vi "Motors Bk 3.vi"(0 "Set":refnum<vi>, 3 "Enable Motors":refnum<vi>, 4 "Scan in Progress":refnum<vi>, 8 "Cluster":T1, 11 "Motors Visa Ref":refnum<visa-resource-name>="COM7") -> ()   [LabVIEW 2010]
uses:
  <vilib>/Utility/error.llb/DialogType.ctl
panel:
  in  "Set Backlash":bool
  out "Motors error":refnum<vi>
  out "theta-":refnum<vi>
  out "theta+":refnum<vi>
  out "Delta Theta (deg)":refnum<vi>
  out "Theta Speed (deg/s)":refnum<vi>
  out "theta-?":refnum<vi>
  out "theta+?":refnum<vi>
  out "Defined Positions":refnum<vi>
  out "Go To Saved Position?":refnum<vi>
  out "Saved Positions":refnum<vi>
  out "z-":refnum<vi>
  out "z+":refnum<vi>
  out "Delta Z (mm)":refnum<vi>
  out "Z Speed (mm/s)":refnum<vi>
  out "z-?":refnum<vi>
  out "z+?":refnum<vi>
  out "Y Speed (mm/s)":refnum<vi>
  out "y-":refnum<vi>
  out "y+":refnum<vi>
  out "Delta Y (mm)":refnum<vi>
  out "y-?":refnum<vi>
  out "y+?":refnum<vi>
  out "x-":refnum<vi>
  out "x+":refnum<vi>
  out "X Speed (mm/s)":refnum<vi>
  out "Delta X (mm)":refnum<vi>
  out "x-?":refnum<vi>
  out "x+?":refnum<vi>
  out "Jog-Mode":refnum<vi>
  out "Theta Go To":refnum<vi>
  out "Theta Go?":refnum<vi>
  out "Z Go To":refnum<vi>
  out "Z Go?":refnum<vi>
  out "Y Go To":refnum<vi>
  out "Y Go?":refnum<vi>
  out "X Go To":refnum<vi>
  out "X Go?":refnum<vi>
  out "Use Datums Nearest Hard Limits to Reset Origin?":refnum<vi>
  out "Saved Limits":refnum<vi>
  out "Find Datums Nearest Hard Limits?":refnum<vi>
  out "Theta Moving":refnum<vi>
  out "Status Theta":refnum<vi>
  out "Theta (deg)":refnum<vi>
  out "Theta Jogger Fast Speed":refnum<vi>
  out "Theta Jogger Normal Speed":refnum<vi>
  out "Theta Slew Speed (mm or degree/s)":refnum<vi>
  out "Z Moving":refnum<vi>
  out "Status Z":refnum<vi>
  out "Z-Axis (mm)":refnum<vi>
  out "Z Jogger Fast Speed":refnum<vi>
  out "Z Jogger Normal Speed":refnum<vi>
  out "Z Slew Speed (mm or degree/s)":refnum<vi>
  out "Y Moving":refnum<vi>
  out "Status Y":refnum<vi>
  out "Y-Axis (mm)":refnum<vi>
  out "Y Jogger Fast Speed":refnum<vi>
  out "Y Jogger Normal Speed":refnum<vi>
  out "Y Slew Speed (mm or degree/s)":refnum<vi>
  out "X Moving":refnum<vi>
  out "Status X":refnum<vi>
  out "X-Axis (mm)":refnum<vi>
  out "X Slew Speed (mm or degree/s)":refnum<vi>
  out "X Jogger Fast Speed":refnum<vi>
  out "X Jogger Normal Speed":refnum<vi>
  out "Set Jogger?":refnum<vi>
  out "Normal":refnum<vi>
  out "Fast":refnum<vi>
  out "Jogger Axis":refnum<vi>
  out "Theta Multiplier":refnum<vi>
  out "Z Multiplier":refnum<vi>
  out "Y Multiplier":refnum<vi>
  out "X Multiplier":refnum<vi>
  out "Need to Update Motor Parameters":refnum<vi>
  out "(degrees/s)":refnum<vi>
  out "Theta Set Slew Speed?":refnum<vi>
  out "(mm/s) 3":refnum<vi>
  out "Z Set Slew Speed?":refnum<vi>
  out "(mm/s) 2":refnum<vi>
  out "Y Set Slew Speed?":refnum<vi>
  out "(mm/s)":refnum<vi>
  out "X Set Slew Speed?":refnum<vi>
  out "Save Current Motor Parameters?":refnum<vi>
  out "Redefine Origin as Current Location?":refnum<vi>
  out "Reset Motors?":refnum<vi>
  out "Manual Communication is Active\n(Close Before Ending Program)":refnum<vi>
  out "Manual IO?":refnum<vi>
  out "EMERGENCY":refnum<vi>
  out "Backlash Theta":refnum<vi>
  out "Backlash Z":refnum<vi>
  out "Backlash Y":refnum<vi>
  out "Backlash X":refnum<vi>
  out "Backlash?":refnum<vi>
  out "Stop Theta?":refnum<vi>
  out "Stop Z?":refnum<vi>
  out "Stop Y?":refnum<vi>
  out "Stop X?":refnum<vi>
  out "Theta Action":string
  out "Z Action":string
  out "Y Action":string
  out "X Action":string
  in  "Steps to deactivate hard limit after finding datums":dbl=1000.0
  out "Loop i":i32
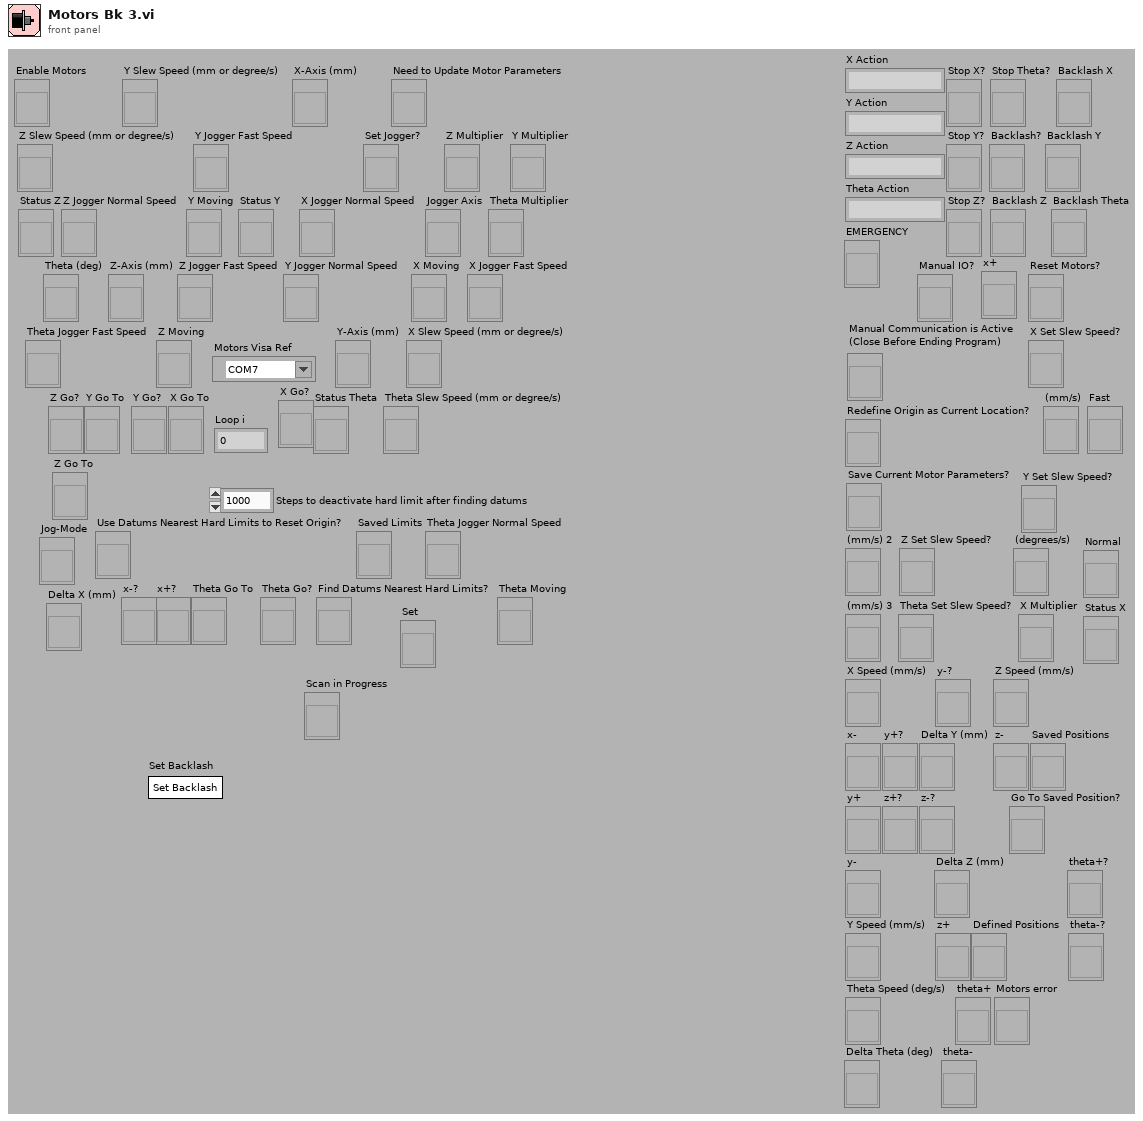
[diagram p1: front panel]
types:
  T1 = cluster{"Stop X?":refnum<vi>, "Stop Y?":refnum<vi>, "Stop Z?":refnum<vi>, "Stop Theta?":refnum<vi>, "Backlash?":refnum<vi>, "Backlash X":refnum<vi>, "Backlash Y":refnum<vi>, "Backlash Z":refnum<vi>, "Backlash Theta":refnum<vi>, "Manual IO?":refnum<vi>, "Manual Communication is Active\n(Close Before Ending Program)":refnum<vi>, "Reset Motors?":refnum<vi>, "Set Jogger?":refnum<vi>, "Normal":refnum<vi>, "Fast":refnum<vi>, "Jogger Axis":refnum<vi>, "Redefine Origin as Current Location?":refnum<vi>, "Save Current Motor Parameters?":refnum<vi>, "Find Datums Nearest Hard Limits?":refnum<vi>, "Saved Limits":refnum<vi>, "Use Datums Nearest Hard Limits to Reset Origin?":refnum<vi>, "X Go?":refnum<vi>, "Y Go?":refnum<vi>, "Z Go?":refnum<vi>, "Theta Go?":refnum<vi>, "Jog-Mode":refnum<vi>, "x+?":refnum<vi>, "x-?":refnum<vi>, "y+?":refnum<vi>, "y-?":refnum<vi>, "z+?":refnum<vi>, "z-?":refnum<vi>, "theta+?":refnum<vi>, "theta-?":refnum<vi>, "X Set Slew Speed?":refnum<vi>, "(mm/s)":refnum<vi>, "Y Set Slew Speed?":refnum<vi>, "(mm/s)":refnum<vi>, "Z Set Slew Speed?":refnum<vi>, "(mm/s)":refnum<vi>, "Theta Set Slew Speed?":refnum<vi>, "(degrees/s)":refnum<vi>, "Go To Saved Position?":refnum<vi>, "Defined Positions":refnum<vi>, "Need to Update Motor Parameters":refnum<vi>, "X Jogger Normal Speed":refnum<vi>, "X Jogger Fast Speed":refnum<vi>, "Y Jogger Normal Speed":refnum<vi>, "Y Jogger Fast Speed":refnum<vi>, "Z Jogger Normal Speed":refnum<vi>, "Z Jogger Fast Speed":refnum<vi>, "Theta Jogger Normal Speed":refnum<vi>, "Theta Jogger Fast Speed":refnum<vi>, "X Moving":refnum<vi>, "Y Moving":refnum<vi>, "Z Moving":refnum<vi>, "Theta Moving":refnum<vi>, "X Slew Speed (mm or degree/s)":refnum<vi>, "Y Slew Speed (mm or degree/s)":refnum<vi>, "Z Slew Speed (mm or degree/s)":refnum<vi>, "Theta Slew Speed (mm or degree/s)":refnum<vi>, "X-Axis (mm)":refnum<vi>, "Y-Axis (mm)":refnum<vi>, "Z-Axis (mm)":refnum<vi>, "Theta (deg)":refnum<vi>, "X Multiplier":refnum<vi>, "Y Multiplier":refnum<vi>, "Z Multiplier":refnum<vi>, "Theta Multiplier":refnum<vi>, "Motors Online":refnum<vi>, "Motors Status":refnum<vi>, "Status X":refnum<vi>, "Status Y":refnum<vi>, "Status Z":refnum<vi>, "Status Theta":refnum<vi>, "Motors error":refnum<vi>, "QUIT":refnum<vi>, "EMERGENCY":refnum<vi>, "X Go To":refnum<vi>, "Y Go To":refnum<vi>, "Z Go To":refnum<vi>, "Theta Go To":refnum<vi>, "Delta X (mm)":refnum<vi>, "Delta Y (mm)":refnum<vi>, "Delta Z (mm)":refnum<vi>, "Delta Theta (deg)":refnum<vi>, "X Speed (mm/s)":refnum<vi>, "Y Speed (mm/s)":refnum<vi>, "Z Speed (mm/s)":refnum<vi>, "Theta Speed (deg/s)":refnum<vi>, "x+":refnum<vi>, "x-":refnum<vi>, "y+":refnum<vi>, "y-":refnum<vi>, "z+":refnum<vi>, "z-":refnum<vi>, "theta+":refnum<vi>, "theta-":refnum<vi>, "Saved Positions":refnum<vi>}
  T2 = typedef "DialogType.ctl" = u16
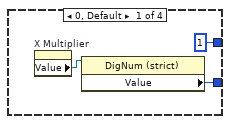
[diagram p4: hidden frame]
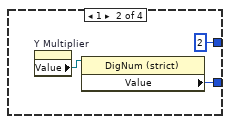
[diagram p5: hidden frame]
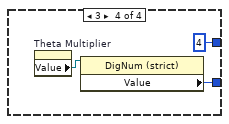
[diagram p6: hidden frame]
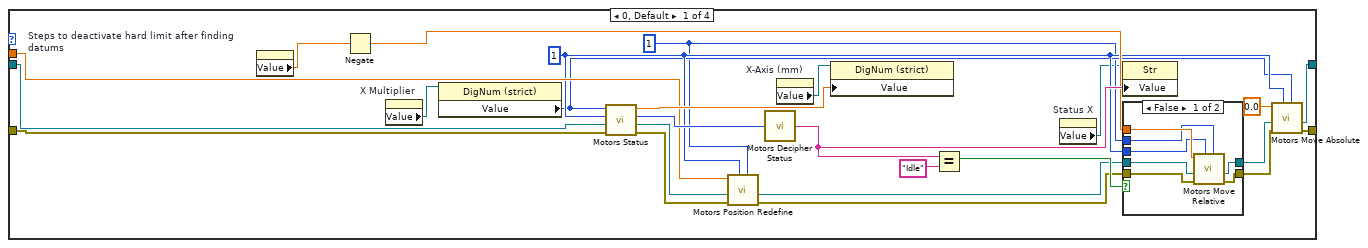
[diagram p16: hidden frame]
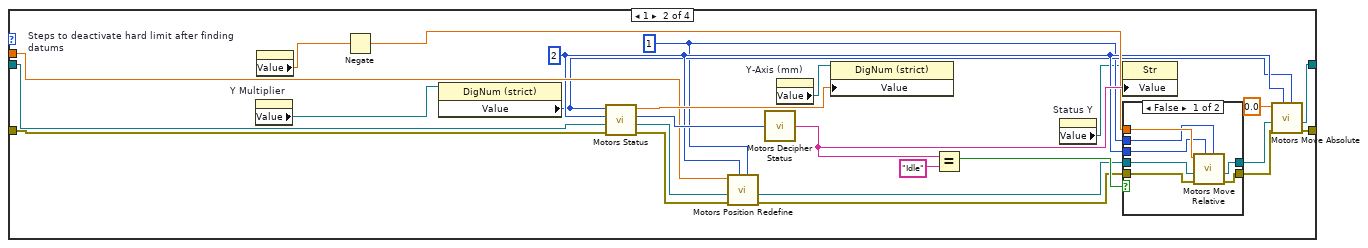
[diagram p18: hidden frame]
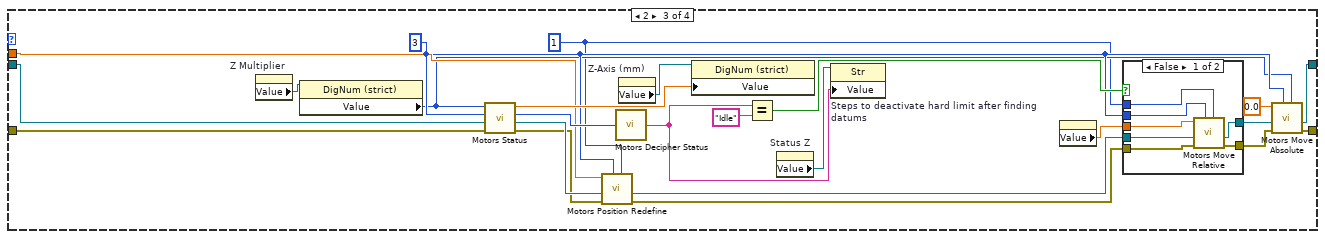
[diagram p20: hidden frame]
diagram:
  w2 = T2 0 items=["no dialog", "OK message", "continue or stop message", "OK message + warnings", "continue/stop + warnings"] ("type of dialog (OK msg:1)")
  n1 = call "Motors Open.vi"("VISA in"="Motors Visa Ref") -> ("error out"=w112:errorcluster, "VISA out"=w4:refnum<visa-resource-name>)  [unwired: 1 in]
  n2 = call <vilib>:"Simple Error Handler.vi"("type of dialog (OK msg:1)"=w2, "error in (no error)"=w112) -> ("error?"=w111:bool, "error out"=w113:errorcluster)  [unwired: 3 in, 3 out]
  n3 = Unbundle("Cluster") -> ("Stop X?"=→"Stop X?":refnum<vi>, "Stop Y?"=→"Stop Y?":refnum<vi>, "Stop Z?"=→"Stop Z?":refnum<vi>, "Stop Theta?"=→"Stop Theta?":refnum<vi>, "Backlash?"=→"Backlash?":refnum<vi>, "Backlash X"=→"Backlash X":refnum<vi>, "Backlash Y"=→"Backlash Y":refnum<vi>, "Backlash Z"=→"Backlash Z":refnum<vi>, "Backlash Theta"=→"Backlash Theta":refnum<vi>, "Manual IO?"=→"Manual IO?":refnum<vi>, "Manual Communication is Active\n(Close Before Ending Program)"=→"Manual Communication is Active\n(Close Before Ending Program)":refnum<vi>, "Reset Motors?"=→"Reset Motors?":refnum<vi>, "Set Jogger?"=→"Set Jogger?":refnum<vi>, "Normal"=→"Normal":refnum<vi>, "Fast"=→"Fast":refnum<vi>, "Jogger Axis"=→"Jogger Axis":refnum<vi>, "Redefine Origin as Current Location?"=→"Redefine Origin as Current Location?":refnum<vi>, "Save Current Motor Parameters?"=→"Save Current Motor Parameters?":refnum<vi>, "Find Datums Nearest Hard Limits?"=→"Find Datums Nearest Hard Limits?":refnum<vi>, "Saved Limits"=→"Saved Limits":refnum<vi>, "Use Datums Nearest Hard Limits to Reset Origin?"=→"Use Datums Nearest Hard Limits to Reset Origin?":refnum<vi>, "X Go?"=→"X Go?":refnum<vi>, "Y Go?"=→"Y Go?":refnum<vi>, "Z Go?"=→"Z Go?":refnum<vi>, "Theta Go?"=→"Theta Go?":refnum<vi>, "Jog-Mode"=→"Jog-Mode":refnum<vi>, "x+?"=→"x+?":refnum<vi>, "x-?"=→"x-?":refnum<vi>, "y+?"=→"y+?":refnum<vi>, "y-?"=→"y-?":refnum<vi>, "z+?"=→"z+?":refnum<vi>, "z-?"=→"z-?":refnum<vi>, "theta+?"=→"theta+?":refnum<vi>, "theta-?"=→"theta-?":refnum<vi>, "X Set Slew Speed?"=→"X Set Slew Speed?":refnum<vi>, "(mm/s)"=→"(mm/s)":refnum<vi>, "Y Set Slew Speed?"=→"Y Set Slew Speed?":refnum<vi>, "(mm/s)"=→"(mm/s) 2":refnum<vi>, "Z Set Slew Speed?"=→"Z Set Slew Speed?":refnum<vi>, "(mm/s)"=→"(mm/s) 3":refnum<vi>, "Theta Set Slew Speed?"=→"Theta Set Slew Speed?":refnum<vi>, "(degrees/s)"=→"(degrees/s)":refnum<vi>, "Go To Saved Position?"=→"Go To Saved Position?":refnum<vi>, "Defined Positions"=→"Defined Positions":refnum<vi>, "Need to Update Motor Parameters"=w7:refnum<vi>, "X Jogger Normal Speed"=→"X Jogger Normal Speed":refnum<vi>, "X Jogger Fast Speed"=→"X Jogger Fast Speed":refnum<vi>, "Y Jogger Normal Speed"=→"Y Jogger Normal Speed":refnum<vi>, "Y Jogger Fast Speed"=→"Y Jogger Fast Speed":refnum<vi>, "Z Jogger Normal Speed"=→"Z Jogger Normal Speed":refnum<vi>, "Z Jogger Fast Speed"=→"Z Jogger Fast Speed":refnum<vi>, "Theta Jogger Normal Speed"=→"Theta Jogger Normal Speed":refnum<vi>, "Theta Jogger Fast Speed"=→"Theta Jogger Fast Speed":refnum<vi>, "X Moving"=→"X Moving":refnum<vi>, "Y Moving"=→"Y Moving":refnum<vi>, "Z Moving"=→"Z Moving":refnum<vi>, "Theta Moving"=→"Theta Moving":refnum<vi>, "X Slew Speed (mm or degree/s)"=→"X Slew Speed (mm or degree/s)":refnum<vi>, "Y Slew Speed (mm or degree/s)"=→"Y Slew Speed (mm or degree/s)":refnum<vi>, "Z Slew Speed (mm or degree/s)"=→"Z Slew Speed (mm or degree/s)":refnum<vi>, "Theta Slew Speed (mm or degree/s)"=→"Theta Slew Speed (mm or degree/s)":refnum<vi>, "X-Axis (mm)"=→"X-Axis (mm)":refnum<vi>, "Y-Axis (mm)"=→"Y-Axis (mm)":refnum<vi>, "Z-Axis (mm)"=→"Z-Axis (mm)":refnum<vi>, "Theta (deg)"=→"Theta (deg)":refnum<vi>, "X Multiplier"=→"X Multiplier":refnum<vi>, "Y Multiplier"=→"Y Multiplier":refnum<vi>, "Z Multiplier"=→"Z Multiplier":refnum<vi>, "Theta Multiplier"=→"Theta Multiplier":refnum<vi>, "Motors Online"=w89:refnum<vi>, "Motors Status"=w90:refnum<vi>, "Status X"=→"Status X":refnum<vi>, "Status Y"=→"Status Y":refnum<vi>, "Status Z"=→"Status Z":refnum<vi>, "Status Theta"=→"Status Theta":refnum<vi>, "Motors error"=w1:refnum<vi>, "QUIT"=w109:refnum<vi>, "EMERGENCY"=→"EMERGENCY":refnum<vi>, "X Go To"=→"X Go To":refnum<vi>, "Y Go To"=→"Y Go To":refnum<vi>, "Z Go To"=→"Z Go To":refnum<vi>, "Theta Go To"=→"Theta Go To":refnum<vi>, "Delta X (mm)"=→"Delta X (mm)":refnum<vi>, "Delta Y (mm)"=→"Delta Y (mm)":refnum<vi>, "Delta Z (mm)"=→"Delta Z (mm)":refnum<vi>, "Delta Theta (deg)"=→"Delta Theta (deg)":refnum<vi>, "X Speed (mm/s)"=→"X Speed (mm/s)":refnum<vi>, "Y Speed (mm/s)"=→"Y Speed (mm/s)":refnum<vi>, "Z Speed (mm/s)"=→"Z Speed (mm/s)":refnum<vi>, "Theta Speed (deg/s)"=→"Theta Speed (deg/s)":refnum<vi>, "x+"=→"x+":refnum<vi>, "x-"=→"x-":refnum<vi>, "y+"=→"y+":refnum<vi>, "y-"=→"y-":refnum<vi>, "z+"=→"z+":refnum<vi>, "z-"=→"z-":refnum<vi>, "theta+"=→"theta+":refnum<vi>, "theta-"=→"theta-":refnum<vi>, "Saved Positions"=→"Saved Positions":refnum<vi>)
  "Need to Update Motor Parameters" <- w7
  "Motors error" <- w1
  n4 = property on="Property Node" class="Clust (strict)"(reference=w1, "Value"=w113) -> ()  [unwired: 1 in, 2 out]
  n5 = property on="Property Node" class="Bool (strict)"(reference=w7, "Value"=TRUE) -> ()  [unwired: 1 in, 2 out]
  n6 = Not(x=w111) -> (.not. x?=w110:bool)
  n7 = property on="Property Node" class="Bool (strict)"(reference=w89, "Value"=w110) -> ()  [unwired: 1 in, 2 out]
  n8 = property on="Property Node" class="Str"(reference=w90, "Value"="Opening Communication Channels") -> (reference out=w108:refnum<vi>)  [unwired: 1 in, 1 out]
  n9 = case shown="True" w110 {
    tunnel: w108 -> [_ w121]
    tunnel: w4 -> [w115 w120]
    tunnel: w1 -> [_ w119]
    tunnel: w109 -> [_ w118]
    tunnel: [w115 w116] -> w3
    frame False {
    }
    frame True {
      n10 = property on="Property Node" class="Str"(reference=w121, "Value"="Running") -> (reference out=w117:refnum<vi>)  [unwired: 1 in, 1 out]
      n11 = while {
        shift-right: [w132] -> w116
        shift-left: w120 -> [w138]
        tunnel: w119 -> [w137]
        tunnel: w118 -> [w140]
        tunnel: w117 -> [w139]
        i -> [w141]
        stop <- w123 stop-if-true
        n12 = property on="Property Node" class="Bool (strict)"(reference="Enable Motors") -> ("Value"=w134:bool)  [unwired: 1 in, 2 out]
        n13 = property on="Property Node" class="Bool (strict)"(reference=w140) -> ("Value"=w136:bool)  [unwired: 1 in, 2 out]
        n14 = property on="Property Node" class="Bool (strict)"(reference="Set") -> (reference out=w126:refnum<vi>, "Value"=w129:bool)  [unwired: 1 in, 1 out]
        n15 = property on="Property Node" class="Bool (strict)"(reference="Scan in Progress") -> ("Value"=w125:bool)  [unwired: 1 in, 2 out]
        n16 = Not(x=w134) -> (.not. x?=w133:bool)
        n17 = Or(x=w136, y=w133) -> (x .or. y?=w124:bool)
        n18 = Or(x=w124, y=w125) -> (x .or. y?=w123:bool)
        n19 = Not(x=w125) -> (.not. x?=w127:bool)
        n20 = Or(x=w129, y=w127) -> (x .or. y?=w131:bool)
        n21 = case shown="True" w131 {
          tunnel: w141 -> [_ w263]
          tunnel: w139 -> [_ w260]
          tunnel: w138 -> [w142 w226]
          tunnel: w137 -> [_ w184]
          tunnel: [w142 w145] -> w132
          tunnel: w126 -> [_ w144]
          frame False {
          }
          frame True {
            # "This loop contains all of the code that has to communicate directly with the manipulator motor controllers.  They are arranged linearly to ensure multiple serial I/O's are never attempted simultaneously.  Note that this loop executes very slowly (each serial I/O takes about 1/20 sec).\n\nWarning: Pushing LabView's \"Clean Up Diagram\" button will likely cause LabView to crash (because this VI is way too big)."
            n22 = property on="Stop X?" class="LVObjRef (strict)"() -> ("Value"=w183:refnum<vi>)  [unwired: 2 in, 2 out]
            n23 = property on="Reset Motors?" class="LVObjRef (strict)"() -> ("Value"=w177:refnum<vi>)  [unwired: 2 in, 2 out]
            n24 = property on="Property Node" class="Bool (strict)"(reference=w144, "Value"=FALSE) -> ()  [unwired: 1 in, 2 out]
            n25 = property on="Property Node" class="Bool (strict)"(reference=w183) -> (reference out=w240:refnum<vi>, "Value"=w233:bool)  [unwired: 1 in, 1 out]
            n26 = property on="Property Node" class="Bool (strict)"(reference=w177) -> (reference out=w220:refnum<vi>, "Value"=w219:bool)  [unwired: 1 in, 1 out]
            n27 = property on="Property Node" class="Clust (strict)"(reference=w184) -> (reference out=w147:refnum<vi>, "Value"=w225:errorcluster)  [unwired: 1 in, 1 out]
            n28 = case shown="True" w233 {
              tunnel: w225 -> [w417 w425]
              tunnel: w226 -> [w418 w424]
              tunnel: [w418 w422] -> w232
              tunnel: [w417 w421] -> w231
              tunnel: w240 -> [_ w419]
              frame False {
              }
              frame True {
                n29 = property on="Property Node" class="Bool (strict)"(reference=w419, "Value"=FALSE) -> ()  [unwired: 1 in, 2 out]
                n30 = call "Motors Stop.vi"("error in"=w425, "Axis"=1, "VISA in"=w424) -> ("error out"=w421:errorcluster, "VISA out"=w422:refnum<visa-resource-name>)
              }
            }
            n31 = property on="Stop Y?" class="LVObjRef (strict)"() -> ("Value"=w182:refnum<vi>)  [unwired: 2 in, 2 out]
            n32 = property on="Property Node" class="Bool (strict)"(reference=w182) -> (reference out=w239:refnum<vi>, "Value"=w234:bool)  [unwired: 1 in, 1 out]
            n33 = case shown="True" w234 {
              tunnel: w231 -> [w408 w416]
              tunnel: w232 -> [w409 w415]
              tunnel: [w409 w413] -> w230
              tunnel: [w408 w412] -> w229
              tunnel: w239 -> [_ w410]
              frame False {
              }
              frame True {
                n34 = property on="Property Node" class="Bool (strict)"(reference=w410, "Value"=FALSE) -> ()  [unwired: 1 in, 2 out]
                n35 = call "Motors Stop.vi"("error in"=w416, "Axis"=2, "VISA in"=w415) -> ("error out"=w412:errorcluster, "VISA out"=w413:refnum<visa-resource-name>)
              }
            }
            n36 = property on="Stop Z?" class="LVObjRef (strict)"() -> ("Value"=w181:refnum<vi>)  [unwired: 2 in, 2 out]
            n37 = property on="Property Node" class="Bool (strict)"(reference=w181) -> (reference out=w238:refnum<vi>, "Value"=w235:bool)  [unwired: 1 in, 1 out]
            n38 = case shown="True" w235 {
              tunnel: w229 -> [w399 w407]
              tunnel: w230 -> [w400 w406]
              tunnel: [w400 w404] -> w228
              tunnel: [w399 w403] -> w227
              tunnel: w238 -> [_ w401]
              frame False {
              }
              frame True {
                n39 = property on="Property Node" class="Bool (strict)"(reference=w401, "Value"=FALSE) -> ()  [unwired: 1 in, 2 out]
                n40 = call "Motors Stop.vi"("error in"=w407, "Axis"=3, "VISA in"=w406) -> ("error out"=w403:errorcluster, "VISA out"=w404:refnum<visa-resource-name>)
              }
            }
            n41 = property on="Stop Theta?" class="LVObjRef (strict)"() -> ("Value"=w180:refnum<vi>)  [unwired: 2 in, 2 out]
            n42 = property on="Property Node" class="Bool (strict)"(reference=w180) -> (reference out=w237:refnum<vi>, "Value"=w236:bool)  [unwired: 1 in, 1 out]
            n43 = case shown="True" w236 {
              tunnel: w227 -> [w390 w398]
              tunnel: w228 -> [w391 w397]
              tunnel: [w391 w395] -> w221
              tunnel: [w390 w394] -> w222
              tunnel: w237 -> [_ w392]
              frame False {
              }
              frame True {
                n44 = property on="Property Node" class="Bool (strict)"(reference=w392, "Value"=FALSE) -> ()  [unwired: 1 in, 2 out]
                n45 = call "Motors Stop.vi"("error in"=w398, "Axis"=4, "VISA in"=w397) -> ("error out"=w394:errorcluster, "VISA out"=w395:refnum<visa-resource-name>)
              }
            }
            n46 = property on="Backlash?" class="LVObjRef (strict)"() -> ("Value"=w179:refnum<vi>)  [unwired: 2 in, 2 out]
            n47 = property on="Property Node" class="Bool (strict)"(reference=w179) -> (reference out=w224:refnum<vi>, "Value"=w223:bool)  [unwired: 1 in, 1 out]
            n48 = case shown="True" w223 {
              tunnel: [w375 w389] -> w214
              tunnel: w224 -> [_ w383]
              tunnel: w221 -> [w375 w382]
              tunnel: w222 -> [w374 w381]
              tunnel: [w374 w380] -> w213
              frame False {
              }
              frame True {
                n49 = property on="Property Node" class="Bool (strict)"(reference=w383, "Value"=FALSE) -> ()  [unwired: 1 in, 2 out]
                n50 = property on="Backlash X" class="LVObjRef (strict)"() -> ("Value"=w379:refnum<vi>)  [unwired: 2 in, 2 out]
                n51 = property on="Backlash Z" class="LVObjRef (strict)"() -> ("Value"=w377:refnum<vi>)  [unwired: 2 in, 2 out]
                n52 = property on="Backlash Y" class="LVObjRef (strict)"() -> ("Value"=w378:refnum<vi>)  [unwired: 2 in, 2 out]
                n53 = property on="Backlash Theta" class="LVObjRef (strict)"() -> ("Value"=w376:refnum<vi>)  [unwired: 2 in, 2 out]
                n54 = property on="Property Node" class="DigNum (strict)"(reference=w379) -> ("Value"=w388:u32)  [unwired: 1 in, 2 out]
                n55 = property on="Property Node" class="DigNum (strict)"(reference=w376) -> ("Value"=w385:u32)  [unwired: 1 in, 2 out]
                n56 = property on="Property Node" class="DigNum (strict)"(reference=w377) -> ("Value"=w386:u32)  [unwired: 1 in, 2 out]
                n57 = property on="Property Node" class="DigNum (strict)"(reference=w378) -> ("Value"=w387:u32)  [unwired: 1 in, 2 out]
                n58 = call "Motors Backlash.vi"("X"=w388, "Y"=w387, "VISA in"=w382, "error in"=w381, "Z"=w386, "Theta"=w385) -> ("VISA out"=w389:refnum<visa-resource-name>, "error out"=w380:errorcluster)  [unwired: 2 in]
              }
            }
            n59 = property on="Manual IO?" class="LVObjRef (strict)"() -> ("Value"=w178:refnum<vi>)  [unwired: 2 in, 2 out]
            n60 = property on="Property Node" class="Bool (strict)"(reference=w178) -> (reference out=w218:refnum<vi>, "Value"=w217:bool)  [unwired: 1 in, 1 out]
            n61 = case shown="True" w217 {
              tunnel: [w349 w360] -> w216
              tunnel: [w350 w352] -> w215
              tunnel: w218 -> [_ w354]
              tunnel: w214 -> [w350 w353]
              tunnel: w213 -> [w349 w351]
              frame False {
              }
              frame True {
                n62 = flat-sequence {
                  tunnel: [w362] -> w356
                  tunnel: [w369] -> w359
                  tunnel: [w368] -> w358
                  tunnel: [w367] -> w357
                  tunnel: w356 -> [w367]
                  tunnel: w353 -> [w366]
                  tunnel: w351 -> [w365]
                  tunnel: [w372] -> w352
                  tunnel: [w373] -> w360
                  tunnel: w359 -> [w373]
                  tunnel: w358 -> [w372]
                  tunnel: w357 -> [w370]
                  frame #0 {
                    n63 = property on="Manual Communication is Active\n(Close Before Ending Program)" class="LVObjRef (strict)"() -> ("Value"=w361:refnum<vi>)  [unwired: 2 in, 2 out]
                    n64 = property on="Property Node" class="Bool (strict)"(reference=w361, "Value"=TRUE ("Manual Communication is Active\n(Close Before Ending Program) 2")) -> (reference out=w362:refnum<vi>)  [unwired: 1 in, 1 out]
                  }
                  frame #1 {
                    n65 = property on="EMERGENCY" class="LVObjRef (strict)"() -> ("Value"=w364:refnum<vi>)  [unwired: 2 in, 2 out]
                    n66 = call "Motors Manual IO.vi"("error in"=w365, "Emergency Stop Reference"=w364, "VISA in"=w366) -> ("error out"=w369:errorcluster, "VISA out"=w368:refnum<visa-resource-name>)
                  }
                  frame #2 {
                    n67 = property on="Property Node" class="Bool (strict)"(reference=w370, "Value"=FALSE ("Manual Communication is Active\n(Close Before Ending Program)")) -> ()  [unwired: 1 in, 2 out]
                  }
                }
                n68 = property on="Property Node" class="Bool (strict)"(reference=w354, "Value"=FALSE) -> ()  [unwired: 1 in, 2 out]
              }
            }
            n69 = property on="Jogger Axis" class="LVObjRef (strict)"() -> ("Value"=w169:refnum<vi>)  [unwired: 2 in, 2 out]
            n70 = property on="Property Node" class="Ring (strict)"(reference=w169) -> ("Value"=w212:u16)  [unwired: 1 in, 2 out]
            n71 = case shown="2" w212 {
              tunnel: [u32 1 u32 2 u32 3 u32 4] -> _
              tunnel: [w315 w318 w321 w324] -> w211
              frame 0, Default {
                n72 = property on="X Multiplier" class="LVObjRef (strict)"() -> ("Value"=w314:refnum<vi>)  [unwired: 2 in, 2 out]
                n73 = property on="Property Node" class="DigNum (strict)"(reference=w314) -> ("Value"=w315:u32)  [unwired: 1 in, 2 out]
              }
              frame 1 {
                n74 = property on="Y Multiplier" class="LVObjRef (strict)"() -> ("Value"=w317:refnum<vi>)  [unwired: 2 in, 2 out]
                n75 = property on="Property Node" class="DigNum (strict)"(reference=w317) -> ("Value"=w318:u32)  [unwired: 1 in, 2 out]
              }
              frame 2 {
                n76 = property on="Z Multiplier" class="LVObjRef (strict)"() -> ("Value"=w320:refnum<vi>)  [unwired: 2 in, 2 out]
                n77 = property on="Property Node" class="DigNum (strict)"(reference=w320) -> ("Value"=w321:u32)  [unwired: 1 in, 2 out]
              }
              frame 3 {
                n78 = property on="Theta Multiplier" class="LVObjRef (strict)"() -> ("Value"=w323:refnum<vi>)  [unwired: 2 in, 2 out]
                n79 = property on="Property Node" class="DigNum (strict)"(reference=w323) -> ("Value"=w324:u32)  [unwired: 1 in, 2 out]
              }
            }
            n80 = case shown="True" w219 {
              tunnel: [w341 w348] -> w207
              tunnel: [w342 w347] -> w208
              tunnel: w215 -> [w342 w346]
              tunnel: w216 -> [w341 w345]
              tunnel: w220 -> [_ w343]
              frame False {
              }
              frame True {
                n81 = property on="Property Node" class="Bool (strict)"(reference=w343, "Value"=FALSE) -> ()  [unwired: 1 in, 2 out]
                n82 = call "Motors Reset.vi"("error in"=w345, "VISA in"=w346) -> ("error out"=w348:errorcluster, "VISA out"=w347:refnum<visa-resource-name>)
              }
            }
            n83 = property on="Set Jogger?" class="LVObjRef (strict)"() -> ("Value"=w170:refnum<vi>)  [unwired: 2 in, 2 out]
            n84 = property on="Property Node" class="Bool (strict)"(reference=w170) -> (reference out=w210:refnum<vi>, "Value"=w209:bool)  [unwired: 1 in, 1 out]
            n85 = case shown="True" w209 {
              tunnel: [w327 w340] -> w205
              tunnel: [w326 w338] -> w206
              tunnel: w211 -> [_ w339]
              tunnel: w210 -> [_ w336]
              tunnel: w207 -> [w327 w332]
              tunnel: w208 -> [w326 w331]
              frame False {
              }
              frame True {
                n86 = property on="Property Node" class="Bool (strict)"(reference=w336, "Value"=FALSE ("Need to Update Motor Parameters")) -> ()  [unwired: 1 in, 2 out]
                n87 = property on="Normal" class="LVObjRef (strict)"() -> ("Value"=w329:refnum<vi>)  [unwired: 2 in, 2 out]
                n88 = property on="Need to Update Motor Parameters" class="LVObjRef (strict)"() -> ("Value"=w328:refnum<vi>)  [unwired: 2 in, 2 out]
                n89 = property on="Fast" class="LVObjRef (strict)"() -> ("Value"=w330:refnum<vi>)  [unwired: 2 in, 2 out]
                n90 = property on="Property Node" class="DigNum (strict)"(reference=w329) -> ("Value"=w335:dbl)  [unwired: 1 in, 2 out]
                n91 = property on="Property Node" class="DigNum (strict)"(reference=w330) -> ("Value"=w334:dbl)  [unwired: 1 in, 2 out]
                n92 = property on="Property Node" class="Bool (strict)"(reference=w328, "Value"=TRUE) -> ()  [unwired: 1 in, 2 out]
                n93 = call "Motors Jogger Speed.vi"("Axis Multiplier"=w339, "error in"=w332, "VISA in"=w331, "Fast Speed (mm or degree/sec)"=w334, "Normal Speed (mm or degree/sec)"=w335) -> ("error out"=w340:errorcluster, "VISA out"=w338:refnum<visa-resource-name>)  [unwired: 5 in]
              }
            }
            n94 = property on="Redefine Origin as Current Location?" class="LVObjRef (strict)"() -> ("Value"=w176:refnum<vi>)  [unwired: 2 in, 2 out]
            n95 = property on="Property Node" class="Bool (strict)"(reference=w176) -> (reference out=w252:refnum<vi>, "Value"=w262:bool)  [unwired: 1 in, 1 out]
            n96 = case shown="True" w262 {
              tunnel: w206 -> [w1424 w1431]
              tunnel: w205 -> [w1425 w1427]
              tunnel: [w1425 w1429] -> w255
              tunnel: [w1424 w1430] -> w313
              tunnel: w252 -> [_ w1426]
              frame False {
              }
              frame True {
                n97 = property on="Property Node" class="Bool (strict)"(reference=w1426, "Value"=FALSE) -> ()  [unwired: 1 in, 2 out]
                n98 = call "Motors Redefine Origin.vi"("error in"=w1427, "VISA in"=w1431) -> ("error out"=w1429:errorcluster, "VISA out"=w1430:refnum<visa-resource-name>)
              }
            }
            n99 = property on="Save Current Motor Parameters?" class="LVObjRef (strict)"() -> ("Value"=w175:refnum<vi>)  [unwired: 2 in, 2 out]
            n100 = property on="Property Node" class="Bool (strict)"(reference=w175) -> (reference out=w254:refnum<vi>, "Value"=w253:bool)  [unwired: 1 in, 1 out]
            n101 = case shown="True" w253 {
              tunnel: w255 -> [w1417 w1423]
              tunnel: [w1417 w1422] -> w269
              tunnel: w313 -> [w1416 w1421]
              tunnel: [w1416 w1420] -> w268
              tunnel: w254 -> [_ w1419]
              frame False {
              }
              frame True {
                n102 = property on="Property Node" class="Bool (strict)"(reference=w1419, "Value"=FALSE) -> ()  [unwired: 1 in, 2 out]
                n103 = call "Motors Save.vi"("error in"=w1423, "VISA in"=w1421) -> ("error out"=w1422:errorcluster, "VISA out"=w1420:refnum<visa-resource-name>)
              }
            }
            n104 = property on="Find Datums Nearest Hard Limits?" class="LVObjRef (strict)"() -> ("Value"=w167:refnum<vi>)  [unwired: 2 in, 2 out]
            n105 = property on="Property Node" class="Bool (strict)"(reference=w167) -> (reference out=w256:refnum<vi>, "Value"=w261:bool)  [unwired: 1 in, 1 out]
            n106 = case shown="True" w261 {
              tunnel: w269 -> [w605 w618]
              tunnel: [w605 w616] -> w266
              tunnel: [w604 w617] -> w264
              tunnel: w268 -> [w604 w619]
              tunnel: w260 -> [w603 w611]
              tunnel: [w603 w608] -> w258
              tunnel: w256 -> [_ w607]
              frame False {
              }
              frame True {
                n107 = property on="Property Node" class="Bool (strict)"(reference=w607, "Value"=FALSE) -> ()  [unwired: 1 in, 2 out]
                n108 = flat-sequence {
                  tunnel: w618 -> [w624]
                  tunnel: w619 -> [w625]
                  tunnel: [w625] -> w615
                  tunnel: [w624] -> w614
                  tunnel: w611 -> [w621]
                  tunnel: [w620] -> w609
                  tunnel: w615 -> [w644]
                  tunnel: w614 -> [w643]
                  tunnel: [w639] -> w613
                  tunnel: [w638] -> w612
                  tunnel: [w628] -> w610
                  tunnel: w609 -> [w628]
                  tunnel: [w738] -> w616
                  tunnel: [w739] -> w617
                  tunnel: w613 -> [w739]
                  tunnel: w612 -> [w738]
                  tunnel: w610 -> [w736]
                  tunnel: [w735] -> w608
                  frame #0 {
                    n109 = call <vilib>:"Set Busy.vi"("disable click? (T)"=FALSE) -> ()  [unwired: 9 in, 2 out]
                    n110 = property on="Property Node" class="Str"(reference=w621, "Value"="Finding Datums Nearest Hard Limits\nThis May Take a Few Minutes" ("Status")) -> (reference out=w620:refnum<vi>)  [unwired: 1 in, 1 out]
                  }
                  frame #1 {
                    n111 = call "Motors Find Datums.vi"("error in"=w643, "VISA in"=w644) -> ("error out"=w640:errorcluster, "VISA out"=w641:refnum<visa-resource-name>)
                    n112 = for {
                      N: 4 -> [_]
                      shift-right: [w648] -> w638
                      shift-left: w640 -> [w649]
                      shift-right: [w647] -> w639
                      shift-left: w641 -> [w650]
                      tunnel: [w646] -> w630 mode=indexing
                      i -> [w645]
                      n113 = case shown="3" w645 {
                        tunnel: w649 -> [w663 w684 w705 w726]
                        tunnel: w650 -> [w664 w685 w706 w727]
                        tunnel: [w657 w678 w698 w719] -> w648
                        tunnel: [w658 w679 w699 w720] -> w647
                        tunnel: [w655 w676 w702 w723] -> w646
                        frame 0, Default {
                          w656 = 1 ("Axis")
                          n114 = property on="X Multiplier" class="LVObjRef (strict)"() -> ("Value"=w651:refnum<vi>)  [unwired: 2 in, 2 out]
                          n115 = property on="Property Node" class="DigNum (strict)"(reference=w651) -> ("Value"=w662:u32)  [unwired: 1 in, 2 out]
                          n116 = call "Motors Status.vi"("error in"=w663, "VISA in"=w664, "Axis"=w656, "Axis Multiplier"=w662) -> ("error out"=w659:errorcluster, "VISA out"=w660:refnum<visa-resource-name>, "OS"=w669:i32, "Actual Position (mm or deg)"=w661:dbl)  [unwired: 3 in]
                          n117 = call "Motors Datum Position.vi"("error in"=w659, "VISA in"=w660, "Axis"=w656) -> ("error out"=w657:errorcluster, "VISA out"=w658:refnum<visa-resource-name>, "Datum Position (steps)"=w655:string)  [unwired: 5 in]
                          n118 = call "Motors Decipher Status.vi"("OS"=w669) -> ("Status"=w668:string)
                          n119 = property on="X-Axis (mm)" class="LVObjRef (strict)"() -> ("Value"=w653:refnum<vi>)  [unwired: 2 in, 2 out]
                          n120 = property on="Property Node" class="DigNum (strict)"(reference=w653, "Value"=w661) -> ()  [unwired: 1 in, 2 out]
                          n121 = Equal?(x=w668, y="Idle") -> (x = y?=w666:bool)
                          n122 = property on="Status X" class="LVObjRef (strict)"() -> ("Value"=w654:refnum<vi>)  [unwired: 2 in, 2 out]
                          n123 = case shown="False" w666 {
                            tunnel: [TRUE FALSE] -> w665
                            frame False {
                            }
                            frame True {
                            }
                          }
                          n124 = property on="Property Node" class="Str"(reference=w654, "Value"=w668) -> ()  [unwired: 1 in, 2 out]
                          n125 = property on="X Moving" class="LVObjRef (strict)"() -> ("Value"=w652:refnum<vi>)  [unwired: 2 in, 2 out]
                          n126 = property on="Property Node" class="Bool (strict)"(reference=w652, "Value"=w665) -> ()  [unwired: 1 in, 2 out]
                        }
                        frame 1 {
                          w677 = 2 ("Axis")
                          n127 = property on="Y Multiplier" class="LVObjRef (strict)"() -> ("Value"=w675:refnum<vi>)  [unwired: 2 in, 2 out]
                          n128 = property on="Property Node" class="DigNum (strict)"(reference=w675) -> ("Value"=w683:u32)  [unwired: 1 in, 2 out]
                          n129 = call "Motors Status.vi"("error in"=w684, "VISA in"=w685, "Axis"=w677, "Axis Multiplier"=w683) -> ("error out"=w680:errorcluster, "VISA out"=w681:refnum<visa-resource-name>, "OS"=w690:i32, "Actual Position (mm or deg)"=w682:dbl)  [unwired: 3 in]
                          n130 = call "Motors Datum Position.vi"("error in"=w680, "VISA in"=w681, "Axis"=w677) -> ("error out"=w678:errorcluster, "VISA out"=w679:refnum<visa-resource-name>, "Datum Position (steps)"=w676:string)  [unwired: 5 in]
                          n131 = call "Motors Decipher Status.vi"("OS"=w690) -> ("Status"=w688:string)
                          n132 = property on="Y-Axis (mm)" class="LVObjRef (strict)"() -> ("Value"=w672:refnum<vi>)  [unwired: 2 in, 2 out]
                          n133 = property on="Property Node" class="DigNum (strict)"(reference=w672, "Value"=w682) -> ()  [unwired: 1 in, 2 out]
                          n134 = Equal?(x=w688, y="Idle") -> (x = y?=w687:bool)
                          n135 = property on="Status Y" class="LVObjRef (strict)"() -> ("Value"=w674:refnum<vi>)  [unwired: 2 in, 2 out]
                          n136 = case shown="False" w687 {
                            tunnel: [TRUE FALSE] -> w686
                            frame False {
                            }
                            frame True {
                            }
                          }
                          n137 = property on="Property Node" class="Str"(reference=w674, "Value"=w688) -> ()  [unwired: 1 in, 2 out]
                          n138 = property on="Y Moving" class="LVObjRef (strict)"() -> ("Value"=w673:refnum<vi>)  [unwired: 2 in, 2 out]
                          n139 = property on="Property Node" class="Bool (strict)"(reference=w673, "Value"=w686) -> ()  [unwired: 1 in, 2 out]
                        }
                        frame 2 {
                          w697 = 3 ("Axis")
                          n140 = property on="Z Multiplier" class="LVObjRef (strict)"() -> ("Value"=w696:refnum<vi>)  [unwired: 2 in, 2 out]
                          n141 = property on="Property Node" class="DigNum (strict)"(reference=w696) -> ("Value"=w704:u32)  [unwired: 1 in, 2 out]
                          n142 = call "Motors Status.vi"("error in"=w705, "VISA in"=w706, "Axis"=w697, "Axis Multiplier"=w704) -> ("error out"=w700:errorcluster, "VISA out"=w701:refnum<visa-resource-name>, "OS"=w711:i32, "Actual Position (mm or deg)"=w703:dbl)  [unwired: 3 in]
                          n143 = call "Motors Datum Position.vi"("error in"=w700, "VISA in"=w701, "Axis"=w697) -> ("error out"=w698:errorcluster, "VISA out"=w699:refnum<visa-resource-name>, "Datum Position (steps)"=w702:string)  [unwired: 5 in]
                          n144 = call "Motors Decipher Status.vi"("OS"=w711) -> ("Status"=w709:string)
                          n145 = property on="Z-Axis (mm)" class="LVObjRef (strict)"() -> ("Value"=w693:refnum<vi>)  [unwired: 2 in, 2 out]
                          n146 = property on="Property Node" class="DigNum (strict)"(reference=w693, "Value"=w703) -> ()  [unwired: 1 in, 2 out]
                          n147 = Equal?(x=w709, y="Idle") -> (x = y?=w708:bool)
                          n148 = property on="Status Z" class="LVObjRef (strict)"() -> ("Value"=w695:refnum<vi>)  [unwired: 2 in, 2 out]
                          n149 = case shown="False" w708 {
                            tunnel: [TRUE FALSE] -> w707
                            frame False {
                            }
                            frame True {
                            }
                          }
                          n150 = property on="Property Node" class="Str"(reference=w695, "Value"=w709) -> ()  [unwired: 1 in, 2 out]
                          n151 = property on="Z Moving" class="LVObjRef (strict)"() -> ("Value"=w694:refnum<vi>)  [unwired: 2 in, 2 out]
                          n152 = property on="Property Node" class="Bool (strict)"(reference=w694, "Value"=w707) -> ()  [unwired: 1 in, 2 out]
                        }
                        frame 3 {
                          w718 = 4 ("Axis")
                          n153 = property on="Theta Multiplier" class="LVObjRef (strict)"() -> ("Value"=w716:refnum<vi>)  [unwired: 2 in, 2 out]
                          n154 = property on="Property Node" class="DigNum (strict)"(reference=w716) -> ("Value"=w725:u32)  [unwired: 1 in, 2 out]
                          n155 = call "Motors Status.vi"("error in"=w726, "VISA in"=w727, "Axis"=w718, "Axis Multiplier"=w725) -> ("error out"=w721:errorcluster, "VISA out"=w722:refnum<visa-resource-name>, "OS"=w732:i32, "Actual Position (mm or deg)"=w724:dbl)  [unwired: 3 in]
                          n156 = call "Motors Datum Position.vi"("error in"=w721, "VISA in"=w722, "Axis"=w718) -> ("error out"=w719:errorcluster, "VISA out"=w720:refnum<visa-resource-name>, "Datum Position (steps)"=w723:string)  [unwired: 5 in]
                          n157 = call "Motors Decipher Status.vi"("OS"=w732) -> ("Status"=w730:string)
                          n158 = property on="Theta (deg)" class="LVObjRef (strict)"() -> ("Value"=w717:refnum<vi>)  [unwired: 2 in, 2 out]
                          n159 = property on="Property Node" class="DigNum (strict)"(reference=w717, "Value"=w724) -> ()  [unwired: 1 in, 2 out]
                          n160 = Equal?(x=w730, y="Idle") -> (x = y?=w729:bool)
                          n161 = property on="Status Theta" class="LVObjRef (strict)"() -> ("Value"=w715:refnum<vi>)  [unwired: 2 in, 2 out]
                          n162 = case shown="True" w729 {
                            tunnel: [TRUE FALSE] -> w728
                            frame False {
                            }
                            frame True {
                            }
                          }
                          n163 = property on="Property Node" class="Str"(reference=w715, "Value"=w730) -> ()  [unwired: 1 in, 2 out]
                          n164 = property on="Theta Moving" class="LVObjRef (strict)"() -> ("Value"=w714:refnum<vi>)  [unwired: 2 in, 2 out]
                          n165 = property on="Property Node" class="Bool (strict)"(reference=w714, "Value"=w728) -> ()  [unwired: 1 in, 2 out]
                        }
                      }
                    }
                    n166 = Build Array (concatenate)("Limits", w630) -> (w629:string[])
                    n167 = Initialize Array("", 0 ("dimension size"), 0 ("dimension size")) -> (w636:string[][])
                    n168 = Build Array (concatenate)(w629, w636) -> (w634:string[][])
                    n169 = property on="Saved Limits" class="LVObjRef (strict)"() -> ("Value"=w626:refnum<vi>)  [unwired: 2 in, 2 out]
                    n170 = property on="Property Node" class="Path"(reference=w626) -> ("Value"=w627:path)  [unwired: 1 in, 2 out]
                    n171 = Transpose 2D Array(2D array=w634) -> (transposed array=w633:string[][])
                    n172 = call "Motors Position Rewrite.vi"("file path"=w627, "Array of Positions"=w633) -> ()  [unwired: 9 in]
                  }
                  frame #2 {
                    n173 = call <vilib>:"Unset Busy.vi"() -> ()  [unwired: 11 in, 1 out]
                    n174 = property on="Property Node" class="Str"(reference=w736, "Value"="Running" ("Status")) -> (reference out=w735:refnum<vi>)  [unwired: 1 in, 1 out]
                  }
                }
              }
            }
            n175 = property on="Use Datums Nearest Hard Limits to Reset Origin?" class="LVObjRef (strict)"() -> ("Value"=w166:refnum<vi>)  [unwired: 2 in, 2 out]
            n176 = property on="Property Node" class="Bool (strict)"(reference=w166) -> (reference out=w146:refnum<vi>, "Value"=w259:bool)  [unwired: 1 in, 1 out]
            n177 = case shown="True" w259 {
              tunnel: [w428 w436] -> w267
              tunnel: w266 -> [w428 w438]
              tunnel: [w427 w435] -> w265
              tunnel: w264 -> [w427 w439]
              tunnel: w258 -> [w426 w431]
              tunnel: [w426 w432] -> w186
              tunnel: w146 -> [_ w430]
              frame False {
              }
              frame True {
                n178 = property on="Property Node" class="Bool (strict)"(reference=w430, "Value"=FALSE) -> ()  [unwired: 1 in, 2 out]
                n179 = flat-sequence {
                  tunnel: w438 -> [w443]
                  tunnel: [w443] -> w437
                  tunnel: w431 -> [w441]
                  tunnel: [w440] -> w433
                  tunnel: w439 -> [w455]
                  tunnel: w437 -> [w456]
                  tunnel: [w451] -> w436
                  tunnel: [w450] -> w435
                  tunnel: [w445] -> w434
                  tunnel: w433 -> [w445]
                  tunnel: w434 -> [w601]
                  tunnel: [w600] -> w432
                  frame #0 {
                    n180 = call <vilib>:"Set Busy.vi"() -> ()  [unwired: 10 in, 2 out]
                    n181 = property on="Property Node" class="Str"(reference=w441, "Value"="Finding Datums Nearest Hard Limits\nThis May Take a Few Minutes" ("Status")) -> (reference out=w440:refnum<vi>)  [unwired: 1 in, 1 out]
                  }
                  frame #1 {
                    n182 = property on="Saved Limits" class="LVObjRef (strict)"() -> ("Value"=w444:refnum<vi>)  [unwired: 2 in, 2 out]
                    n183 = property on="Property Node" class="Path"(reference=w444) -> ("Value"=w446:path)  [unwired: 1 in, 2 out]
                    n184 = call "Motors Find Datums.vi"("error in"=w456, "VISA in"=w455) -> ("error out"=w453:errorcluster, "VISA out"=w454:refnum<visa-resource-name>)
                    n185 = call "Motors Position Load.vi"("error in"=w453, "file path"=w446) -> ("error out"=w452:errorcluster, "Positions"=w449:string[][])
                    n186 = Delete From Array(array=w449, index (row)=0) -> (array with subset deleted=w447:string[][])  [unwired: 2 in, 1 out]
                    n187 = for {
                      shift-right: [w463] -> w451
                      shift-left: w452 -> [w464]
                      shift-right: [w462] -> w450
                      shift-left: w454 -> [w465]
                      tunnel: w447 -> [w461] mode=indexing
                      i -> [w458]
                      n188 = Index Array(array=w461, index=0) -> (element=w460:string)
                      n189 = Fract/Exp String To Number(string=w460) -> (number=w459:dbl)  [unwired: 3 in, 1 out]
                      n190 = case shown="3" w458 {
                        tunnel: w464 -> [w485 w519 w549 w585]
                        tunnel: w465 -> [w486 w520 w550 w586]
                        tunnel: [w479 w512 w541 w578] -> w463
                        tunnel: [w480 w513 w542 w579] -> w462
                        tunnel: w459 -> [w481 w515 w552 w581]
                        frame 0, Default {
                          w469 = u32 1 ("Axis Multiplier")
                          w471 = 1 ("Axis")
                          n191 = property on="Steps to deactivate hard limit after finding datums" class="DigNum (strict)"() -> ("Value"=w477:dbl)  [unwired: 2 in, 2 out]
                          n192 = Negate(x=w477) -> (-x=w472:dbl)
                          n193 = property on="X Multiplier" class="LVObjRef (strict)"() -> ("Value"=w467:refnum<vi>)  [unwired: 2 in, 2 out]
                          n194 = property on="Property Node" class="DigNum (strict)"(reference=w467) -> ("Value"=w470:u32)  [unwired: 1 in, 2 out]
                          n195 = call "Motors Status.vi"("error in"=w485, "VISA in"=w486, "Axis"=w471, "Axis Multiplier"=w470) -> ("error out"=w482:errorcluster, "VISA out"=w483:refnum<visa-resource-name>, "OS"=w490:i32, "Actual Position (mm or deg)"=w484:dbl)  [unwired: 3 in]
                          n196 = call "Motors Position Redefine.vi"("Axis Multiplier"=w469, "Axis"=w471, "error in"=w482, "VISA in"=w483, "Position (mm or deg)"=w481) -> ("error out"=w476:errorcluster, "VISA out"=w473:refnum<visa-resource-name>)  [unwired: 5 in]
                          n197 = call "Motors Decipher Status.vi"("OS"=w490) -> ("Status"=w489:string)
                          n198 = property on="X-Axis (mm)" class="LVObjRef (strict)"() -> ("Value"=w466:refnum<vi>)  [unwired: 2 in, 2 out]
                          n199 = property on="Property Node" class="DigNum (strict)"(reference=w466, "Value"=w484) -> ()  [unwired: 1 in, 2 out]
                          n200 = Equal?(x=w489, y="Idle") -> (x = y?=w487:bool)
                          n201 = property on="Status X" class="LVObjRef (strict)"() -> ("Value"=w468:refnum<vi>)  [unwired: 2 in, 2 out]
                          n202 = property on="Property Node" class="Str"(reference=w468, "Value"=w489) -> ()  [unwired: 1 in, 2 out]
                          n203 = case shown="False" w487 {
                            tunnel: w476 -> [w497 w499]
                            tunnel: [w496 w499] -> w475
                            tunnel: w473 -> [w495 w498]
                            tunnel: [w494 w498] -> w474
                            tunnel: w472 -> [w493 _]
                            tunnel: w471 -> [w492 _]
                            tunnel: w469 -> [w491 _]
                            frame False {
                              n204 = call "Motors Move Relative.vi"("Axis Multiplier"=w491, "Axis"=w492, "error in"=w497, "VISA in"=w495, "Distance (mm)"=w493) -> ("error out"=w496:errorcluster, "VISA out"=w494:refnum<visa-resource-name>)  [unwired: 5 in]
                            }
                            frame True {
                            }
                          }
                          n205 = call "Motors Move Absolute.vi"("Axis Multiplier"=w470, "Axis"=w471, "error in"=w475, "VISA in"=w474, "Position (mm or degree)"=0.0) -> ("error out"=w479:errorcluster, "VISA out"=w480:refnum<visa-resource-name>)  [unwired: 5 in]
                        }
                        frame 1 {
                          w503 = u32 1 ("Axis Multiplier")
                          w505 = 2 ("Axis")
                          n206 = property on="Y Multiplier" class="LVObjRef (strict)"() -> ("Value"=w502:refnum<vi>)  [unwired: 2 in, 2 out]
                          n207 = property on="Steps to deactivate hard limit after finding datums" class="DigNum (strict)"() -> ("Value"=w511:dbl)  [unwired: 2 in, 2 out]
                          n208 = Negate(x=w511) -> (-x=w506:dbl)
                          n209 = property on="Property Node" class="DigNum (strict)"(reference=w502) -> ("Value"=w504:u32)  [unwired: 1 in, 2 out]
                          n210 = call "Motors Status.vi"("error in"=w519, "VISA in"=w520, "Axis"=w505, "Axis Multiplier"=w504) -> ("error out"=w516:errorcluster, "VISA out"=w517:refnum<visa-resource-name>, "OS"=w524:i32, "Actual Position (mm or deg)"=w518:dbl)  [unwired: 3 in]
                          n211 = call "Motors Position Redefine.vi"("Axis Multiplier"=w503, "Axis"=w505, "error in"=w516, "VISA in"=w517, "Position (mm or deg)"=w515) -> ("error out"=w509:errorcluster, "VISA out"=w510:refnum<visa-resource-name>)  [unwired: 5 in]
                          n212 = call "Motors Decipher Status.vi"("OS"=w524) -> ("Status"=w522:string)
                          n213 = property on="Y-Axis (mm)" class="LVObjRef (strict)"() -> ("Value"=w500:refnum<vi>)  [unwired: 2 in, 2 out]
                          n214 = property on="Property Node" class="DigNum (strict)"(reference=w500, "Value"=w518) -> ()  [unwired: 1 in, 2 out]
                          n215 = Equal?(x=w522, y="Idle") -> (x = y?=w521:bool)
                          n216 = property on="Status Y" class="LVObjRef (strict)"() -> ("Value"=w501:refnum<vi>)  [unwired: 2 in, 2 out]
                          n217 = property on="Property Node" class="Str"(reference=w501, "Value"=w522) -> ()  [unwired: 1 in, 2 out]
                          n218 = case shown="False" w521 {
                            tunnel: w510 -> [w531 w532]
                            tunnel: w509 -> [w530 w533]
                            tunnel: [w529 w532] -> w508
                            tunnel: [w528 w533] -> w507
                            tunnel: w506 -> [w527 _]
                            tunnel: w505 -> [w526 _]
                            tunnel: w503 -> [w525 _]
                            frame False {
                              n219 = call "Motors Move Relative.vi"("Axis Multiplier"=w525, "Axis"=w526, "error in"=w530, "VISA in"=w531, "Distance (mm)"=w527) -> ("error out"=w528:errorcluster, "VISA out"=w529:refnum<visa-resource-name>)  [unwired: 5 in]
                            }
                            frame True {
                            }
                          }
                          n220 = call "Motors Move Absolute.vi"("Axis Multiplier"=w504, "Axis"=w505, "error in"=w507, "VISA in"=w508, "Position (mm or degree)"=0.0) -> ("error out"=w512:errorcluster, "VISA out"=w513:refnum<visa-resource-name>)  [unwired: 5 in]
                        }
                        frame 2 {
                          w537 = u32 1 ("Axis Multiplier")
                          w539 = 3 ("Axis")
                          n221 = property on="Z Multiplier" class="LVObjRef (strict)"() -> ("Value"=w535:refnum<vi>)  [unwired: 2 in, 2 out]
                          n222 = property on="Property Node" class="DigNum (strict)"(reference=w535) -> ("Value"=w538:u32)  [unwired: 1 in, 2 out]
                          n223 = call "Motors Status.vi"("error in"=w549, "VISA in"=w550, "Axis"=w539, "Axis Multiplier"=w538) -> ("error out"=w547:errorcluster, "VISA out"=w548:refnum<visa-resource-name>, "OS"=w557:i32, "Actual Position (mm or deg)"=w553:dbl)  [unwired: 3 in]
                          n224 = call "Motors Position Redefine.vi"("Axis Multiplier"=w537, "Axis"=w539, "error in"=w547, "VISA in"=w548, "Position (mm or deg)"=w552) -> ("error out"=w545:errorcluster, "VISA out"=w546:refnum<visa-resource-name>)  [unwired: 5 in]
                          n225 = call "Motors Decipher Status.vi"("OS"=w557) -> ("Status"=w555:string)
                          n226 = property on="Z-Axis (mm)" class="LVObjRef (strict)"() -> ("Value"=w534:refnum<vi>)  [unwired: 2 in, 2 out]
                          n227 = property on="Property Node" class="DigNum (strict)"(reference=w534, "Value"=w553) -> ()  [unwired: 1 in, 2 out]
                          n228 = Equal?(x=w555, y="Idle") -> (x = y?=w554:bool)
                          n229 = property on="Status Z" class="LVObjRef (strict)"() -> ("Value"=w536:refnum<vi>)  [unwired: 2 in, 2 out]
                          n230 = property on="Property Node" class="Str"(reference=w536, "Value"=w555) -> ()  [unwired: 1 in, 2 out]
                          n231 = property on="Steps to deactivate hard limit after finding datums" class="DigNum (strict)"() -> ("Value"=w540:dbl)  [unwired: 2 in, 2 out]
                          n232 = case shown="False" w554 {
                            tunnel: w546 -> [w564 w565]
                            tunnel: w545 -> [w563 w566]
                            tunnel: [w562 w565] -> w544
                            tunnel: [w561 w566] -> w543
                            tunnel: w540 -> [w560 _]
                            tunnel: w539 -> [w559 _]
                            tunnel: w537 -> [w558 _]
                            frame False {
                              n233 = call "Motors Move Relative.vi"("Axis Multiplier"=w558, "Axis"=w559, "error in"=w563, "VISA in"=w564, "Distance (mm)"=w560) -> ("error out"=w561:errorcluster, "VISA out"=w562:refnum<visa-resource-name>)  [unwired: 5 in]
                            }
                            frame True {
                            }
                          }
                          n234 = call "Motors Move Absolute.vi"("Axis Multiplier"=w538, "Axis"=w539, "error in"=w543, "VISA in"=w544, "Position (mm or degree)"=0.0) -> ("error out"=w541:errorcluster, "VISA out"=w542:refnum<visa-resource-name>)  [unwired: 5 in]
                        }
                        frame 3 {
                          w570 = u32 1 ("Axis Multiplier")
                          w572 = 4 ("Axis")
                          n235 = property on="Theta Multiplier" class="LVObjRef (strict)"() -> ("Value"=w568:refnum<vi>)  [unwired: 2 in, 2 out]
                          n236 = property on="Property Node" class="DigNum (strict)"(reference=w568) -> ("Value"=w571:u32)  [unwired: 1 in, 2 out]
                          n237 = call "Motors Status.vi"("error in"=w585, "VISA in"=w586, "Axis"=w572, "Axis Multiplier"=w571) -> ("error out"=w582:errorcluster, "VISA out"=w583:refnum<visa-resource-name>, "OS"=w590:i32, "Actual Position (mm or deg)"=w584:dbl)  [unwired: 3 in]
                          n238 = call "Motors Position Redefine.vi"("Axis Multiplier"=w570, "Axis"=w572, "error in"=w582, "VISA in"=w583, "Position (mm or deg)"=w581) -> ("error out"=w576:errorcluster, "VISA out"=w577:refnum<visa-resource-name>)  [unwired: 5 in]
                          n239 = call "Motors Decipher Status.vi"("OS"=w590) -> ("Status"=w588:string)
                          n240 = property on="Theta (deg)" class="LVObjRef (strict)"() -> ("Value"=w567:refnum<vi>)  [unwired: 2 in, 2 out]
                          n241 = property on="Property Node" class="DigNum (strict)"(reference=w567, "Value"=w584) -> ()  [unwired: 1 in, 2 out]
                          n242 = Equal?(x=w588, y="Idle") -> (x = y?=w587:bool)
                          n243 = property on="Status Theta" class="LVObjRef (strict)"() -> ("Value"=w569:refnum<vi>)  [unwired: 2 in, 2 out]
                          n244 = property on="Property Node" class="Str"(reference=w569, "Value"=w588) -> ()  [unwired: 1 in, 2 out]
                          n245 = case shown="False" w587 {
                            tunnel: w577 -> [w597 w599]
                            tunnel: w576 -> [w596 w598]
                            tunnel: [w595 w599] -> w575
                            tunnel: [w594 w598] -> w574
                            tunnel: "Steps to deactivate hard limit after finding datums" -> [w593 _]
                            tunnel: w572 -> [w592 _]
                            tunnel: w570 -> [w591 _]
                            frame False {
                              n246 = call "Motors Move Relative.vi"("Axis Multiplier"=w591, "Axis"=w592, "error in"=w596, "VISA in"=w597, "Distance (mm)"=w593) -> ("error out"=w594:errorcluster, "VISA out"=w595:refnum<visa-resource-name>)  [unwired: 5 in]
                            }
                            frame True {
                            }
                          }
                          n247 = call "Motors Move Absolute.vi"("Axis Multiplier"=w571, "Axis"=w572, "error in"=w574, "VISA in"=w575, "Position (mm or degree)"=0.0) -> ("error out"=w578:errorcluster, "VISA out"=w579:refnum<visa-resource-name>)  [unwired: 5 in]
                        }
                      }
                    }
                  }
                  frame #2 {
                    n248 = call <vilib>:"Unset Busy.vi"() -> ()  [unwired: 11 in, 1 out]
                    n249 = property on="Property Node" class="Str"(reference=w601, "Value"="Running" ("Status")) -> (reference out=w600:refnum<vi>)  [unwired: 1 in, 1 out]
                  }
                }
              }
            }
            n250 = property on="X Go?" class="LVObjRef (strict)"() -> ("Value"=w165:refnum<vi>)  [unwired: 2 in, 2 out]
            n251 = property on="Property Node" class="Bool (strict)"(reference=w165) -> (reference out=w245:refnum<vi>, "Value"=w257:bool)  [unwired: 1 in, 1 out]
            n252 = case shown="True" w257 {
              tunnel: w265 -> [w1404 w1412]
              tunnel: w267 -> [w1403 w1415]
              tunnel: [w1404 w1413] -> w312
              tunnel: [w1403 w1414] -> w311
              tunnel: w245 -> [_ w1410]
              frame False {
              }
              frame True {
                n253 = property on="Property Node" class="Bool (strict)"(reference=w1410, "Value"=FALSE) -> ()  [unwired: 1 in, 2 out]
                n254 = property on="X Go To" class="LVObjRef (strict)"() -> ("Value"=w1405:refnum<vi>)  [unwired: 2 in, 2 out]
                n255 = property on="X Multiplier" class="LVObjRef (strict)"() -> ("Value"=w1406:refnum<vi>)  [unwired: 2 in, 2 out]
                n256 = property on="Property Node" class="DigNum (strict)"(reference=w1405) -> ("Value"=w1407:dbl)  [unwired: 1 in, 2 out]
                n257 = property on="Property Node" class="DigNum (strict)"(reference=w1406) -> ("Value"=w1408:u32)  [unwired: 1 in, 2 out]
                n258 = call "Motors Move Absolute.vi"("Axis Multiplier"=w1408, "Axis"=u32 1, "error in"=w1415, "VISA in"=w1412, "Position (mm or degree)"=w1407) -> ("error out"=w1414:errorcluster, "VISA out"=w1413:refnum<visa-resource-name>)  [unwired: 5 in]
              }
            }
            n259 = property on="Y Go?" class="LVObjRef (strict)"() -> ("Value"=w164:refnum<vi>)  [unwired: 2 in, 2 out]
            n260 = property on="Property Node" class="Bool (strict)"(reference=w164) -> (reference out=w250:refnum<vi>, "Value"=w251:bool)  [unwired: 1 in, 1 out]
            n261 = case shown="True" w251 {
              tunnel: w312 -> [w1391 w1399]
              tunnel: w311 -> [w1390 w1402]
              tunnel: [w1391 w1400] -> w310
              tunnel: [w1390 w1401] -> w309
              tunnel: w250 -> [_ w1394]
              frame False {
              }
              frame True {
                n262 = property on="Property Node" class="Bool (strict)"(reference=w1394, "Value"=FALSE) -> ()  [unwired: 1 in, 2 out]
                n263 = property on="Y Go To" class="LVObjRef (strict)"() -> ("Value"=w1393:refnum<vi>)  [unwired: 2 in, 2 out]
                n264 = property on="Y Multiplier" class="LVObjRef (strict)"() -> ("Value"=w1392:refnum<vi>)  [unwired: 2 in, 2 out]
                n265 = property on="Property Node" class="DigNum (strict)"(reference=w1392) -> ("Value"=w1397:u32)  [unwired: 1 in, 2 out]
                n266 = property on="Property Node" class="DigNum (strict)"(reference=w1393) -> ("Value"=w1396:dbl)  [unwired: 1 in, 2 out]
                n267 = call "Motors Move Absolute.vi"("Axis Multiplier"=w1397, "Axis"=u32 2, "error in"=w1402, "VISA in"=w1399, "Position (mm or degree)"=w1396) -> ("error out"=w1401:errorcluster, "VISA out"=w1400:refnum<visa-resource-name>)  [unwired: 5 in]
              }
            }
            n268 = property on="Z Go?" class="LVObjRef (strict)"() -> ("Value"=w163:refnum<vi>)  [unwired: 2 in, 2 out]
            n269 = property on="Property Node" class="Bool (strict)"(reference=w163) -> (reference out=w248:refnum<vi>, "Value"=w249:bool)  [unwired: 1 in, 1 out]
            n270 = case shown="True" w249 {
              tunnel: w310 -> [w1378 w1384]
              tunnel: w309 -> [w1377 w1389]
              tunnel: [w1378 w1387] -> w308
              tunnel: [w1377 w1388] -> w307
              tunnel: w248 -> [_ w1381]
              frame False {
              }
              frame True {
                n271 = property on="Property Node" class="Bool (strict)"(reference=w1381, "Value"=FALSE) -> ()  [unwired: 1 in, 2 out]
                n272 = property on="Z Go To" class="LVObjRef (strict)"() -> ("Value"=w1380:refnum<vi>)  [unwired: 2 in, 2 out]
                n273 = property on="Z Multiplier" class="LVObjRef (strict)"() -> ("Value"=w1379:refnum<vi>)  [unwired: 2 in, 2 out]
                n274 = property on="Property Node" class="DigNum (strict)"(reference=w1379) -> ("Value"=w1385:u32)  [unwired: 1 in, 2 out]
                n275 = property on="Property Node" class="DigNum (strict)"(reference=w1380) -> ("Value"=w1383:dbl)  [unwired: 1 in, 2 out]
                n276 = call "Motors Move Absolute.vi"("Axis Multiplier"=w1385, "Axis"=u32 3, "error in"=w1389, "VISA in"=w1384, "Position (mm or degree)"=w1383) -> ("error out"=w1388:errorcluster, "VISA out"=w1387:refnum<visa-resource-name>)  [unwired: 5 in]
              }
            }
            n277 = property on="Theta Go?" class="LVObjRef (strict)"() -> ("Value"=w162:refnum<vi>)  [unwired: 2 in, 2 out]
            n278 = property on="Property Node" class="Bool (strict)"(reference=w162) -> (reference out=w246:refnum<vi>, "Value"=w247:bool)  [unwired: 1 in, 1 out]
            n279 = case shown="True" w247 {
              tunnel: w308 -> [w1364 w1373]
              tunnel: w307 -> [w1365 w1376]
              tunnel: [w1365 w1375] -> w305
              tunnel: [w1364 w1374] -> w306
              tunnel: w246 -> [_ w1368]
              frame False {
              }
              frame True {
                n280 = property on="Property Node" class="Bool (strict)"(reference=w1368, "Value"=FALSE) -> ()  [unwired: 1 in, 2 out]
                n281 = property on="Theta Multiplier" class="LVObjRef (strict)"() -> ("Value"=w1366:refnum<vi>)  [unwired: 2 in, 2 out]
                n282 = property on="Theta Go To" class="LVObjRef (strict)"() -> ("Value"=w1367:refnum<vi>)  [unwired: 2 in, 2 out]
                n283 = property on="Property Node" class="DigNum (strict)"(reference=w1366) -> ("Value"=w1371:u32)  [unwired: 1 in, 2 out]
                n284 = property on="Property Node" class="DigNum (strict)"(reference=w1367) -> ("Value"=w1370:dbl)  [unwired: 1 in, 2 out]
                n285 = call "Motors Move Absolute.vi"("Axis Multiplier"=w1371, "Axis"=u32 4, "error in"=w1376, "VISA in"=w1373, "Position (mm or degree)"=w1370) -> ("error out"=w1375:errorcluster, "VISA out"=w1374:refnum<visa-resource-name>)  [unwired: 5 in]
              }
            }
            n286 = property on="x+?" class="LVObjRef (strict)"() -> ("Value"=w160:refnum<vi>)  [unwired: 2 in, 2 out]
            n287 = property on="x-?" class="LVObjRef (strict)"() -> ("Value"=w159:refnum<vi>)  [unwired: 2 in, 2 out]
            n288 = property on="Property Node" class="Bool (strict)"(reference=w160) -> (reference out=w243:refnum<vi>, "Value"=w277:bool)  [unwired: 1 in, 1 out]
            n289 = property on="Property Node" class="Bool (strict)"(reference=w159) -> (reference out=w244:refnum<vi>, "Value"=w276:bool)  [unwired: 1 in, 1 out]
            n290 = property on="Jog-Mode" class="LVObjRef (strict)"() -> ("Value"=w161:refnum<vi>)  [unwired: 2 in, 2 out]
            n291 = property on="Property Node" class="Bool (strict)"(reference=w161) -> ("Value"=w203:bool)  [unwired: 1 in, 2 out]
            n292 = Or(x=w277, y=w276) -> (x .or. y?=w304:bool)
            n293 = case shown="True" w304 {
              tunnel: w306 -> [w1276 w1286]
              tunnel: w305 -> [w1275 w1285]
              tunnel: w203 -> [_ w1287]
              tunnel: [w1276 w1283] -> w303
              tunnel: [w1275 w1282] -> w302
              tunnel: w276 -> [_ w1284]
              tunnel: w244 -> [_ w1279]
              tunnel: w243 -> [_ w1278]
              frame False {
              }
              frame True {
                n294 = property on="X Multiplier" class="LVObjRef (strict)"() -> ("Value"=w1277:refnum<vi>)  [unwired: 2 in, 2 out]
                n295 = flat-sequence {
                  tunnel: w1287 -> [w1294]
                  tunnel: w1286 -> [w1293]
                  tunnel: w1285 -> [w1292]
                  tunnel: w1284 -> [w1291]
                  tunnel: [w1290] -> w1281
                  tunnel: [w1289] -> w1280
                  tunnel: w1277 -> [w1288]
                  tunnel: [w1362] -> w1282
                  tunnel: [w1363] -> w1283
                  tunnel: w1281 -> [w1363]
                  tunnel: w1280 -> [w1362]
                  tunnel: w1279 -> [w1359]
                  tunnel: w1278 -> [w1358]
                  frame #0 {
                    n296 = case shown="True" w1294 {
                      tunnel: w1293 -> [w1303 w1329]
                      tunnel: w1292 -> [w1299 w1332]
                      tunnel: w1291 -> [w1302 w1337]
                      tunnel: [w1301 w1334] -> w1290
                      tunnel: [w1300 w1333] -> w1289
                      tunnel: w1288 -> [w1296 w1324]
                      frame False {
                        n297 = property on="X Moving" class="LVObjRef (strict)"() -> ("Value"=w1295:refnum<vi>)  [unwired: 2 in, 2 out]
                        n298 = property on="Property Node" class="Bool (strict)"(reference=w1295) -> (reference out=w1297:refnum<vi>, "Value"=w1298:bool)  [unwired: 1 in, 1 out]
                        n299 = case shown="False" w1298 {
                          tunnel: w1303 -> [w1311 w1322]
                          tunnel: w1299 -> [w1316 w1321]
                          tunnel: w1302 -> [w1315 _]
                          tunnel: [w1313 w1322] -> w1301
                          tunnel: [w1314 w1321] -> w1300
                          tunnel: w1297 -> [w1307 _]
                          tunnel: w1296 -> [w1305 _]
                          frame False {
                            n300 = property on="Delta X (mm)" class="LVObjRef (strict)"() -> ("Value"=w1304:refnum<vi>)  [unwired: 2 in, 2 out]
                            n301 = property on="Property Node" class="DigNum (strict)"(reference=w1304) -> ("Value"=w1306:dbl)  [unwired: 1 in, 2 out]
                            n302 = property on="Property Node" class="Bool (strict)"(reference=w1307, "Value"=TRUE ("X Moving")) -> ()  [unwired: 1 in, 2 out]
                            n303 = property on="Property Node" class="DigNum (strict)"(reference=w1305) -> ("Value"=w1309:u32)  [unwired: 1 in, 2 out]
                            n304 = case shown="True" w1315 {
                              tunnel: w1306 -> [w1317 w1319]
                              tunnel: [w1317 w1318] -> w1312
                              frame False {
                              }
                              frame True {
                                n305 = Multiply(x=w1319, y=-1.0) -> (x*y=w1318:dbl)
                              }
                            }
                            n306 = call "Motors Move Relative.vi"("Axis Multiplier"=w1309, "Axis"=1, "error in"=w1316, "VISA in"=w1311, "Distance (mm)"=w1312) -> ("error out"=w1314:errorcluster, "VISA out"=w1313:refnum<visa-resource-name>)  [unwired: 5 in]
                          }
                          frame True {
                          }
                        }
                      }
                      frame True {
                        w1326 = 1 ("Axis")
                        n307 = property on="Property Node" class="DigNum (strict)"(reference=w1324) -> ("Value"=w1327:u32)  [unwired: 1 in, 2 out]
                        n308 = property on="X Speed (mm/s)" class="LVObjRef (strict)"() -> ("Value"=w1323:refnum<vi>)  [unwired: 2 in, 2 out]
                        n309 = property on="Property Node" class="DigNum (strict)"(reference=w1323) -> ("Value"=w1325:dbl)  [unwired: 1 in, 2 out]
                        n310 = case shown="True" w1337 {
                          tunnel: w1325 -> [w1354 w1356]
                          tunnel: [w1354 w1355] -> w1330
                          frame False {
                          }
                          frame True {
                            n311 = Multiply(x=w1356, y=-1.0) -> (x*y=w1355:dbl)
                          }
                        }
                        n312 = call "Motors Move Constant Velocity.vi"("Axis Multiplier"=w1327, "Axis"=w1326, "error in"=w1332, "VISA in"=w1329, "Speed (mm/s)"=w1330) -> ("error out"=w1331:errorcluster, "VISA out"=w1328:refnum<visa-resource-name>)  [unwired: 5 in]
                        n313 = while {
                          tunnel: w1328 -> [w1343]
                          tunnel: [w1345] -> w1336
                          tunnel: w1331 -> [w1346]
                          tunnel: [w1344] -> w1335
                          tunnel: w1327 -> [w1342]
                          stop <- w1351 continue-if-true
                          n314 = property on="x+" class="LVObjRef (strict)"() -> ("Value"=w1338:refnum<vi>)  [unwired: 2 in, 2 out]
                          n315 = property on="x-" class="LVObjRef (strict)"() -> ("Value"=w1339:refnum<vi>)  [unwired: 2 in, 2 out]
                          n316 = property on="Property Node" class="Bool (strict)"(reference=w1338) -> ("Value"=w1352:bool)  [unwired: 1 in, 2 out]
                          n317 = property on="Property Node" class="Bool (strict)"(reference=w1339) -> ("Value"=w1353:bool)  [unwired: 1 in, 2 out]
                          n318 = call "Motors Status.vi"("error in"=w1346, "VISA in"=w1343, "Axis"=1, "Axis Multiplier"=w1342) -> ("error out"=w1344:errorcluster, "VISA out"=w1345:refnum<visa-resource-name>, "OS"=w1349:i32, "Actual Position (mm or deg)"=w1347:dbl)  [unwired: 3 in]
                          n319 = Or(x=w1352, y=w1353) -> (x .or. y?=w1351:bool)
                          n320 = call "Motors Decipher Status.vi"("OS"=w1349) -> ("Status"=w1348:string)
                          n321 = property on="X-Axis (mm)" class="LVObjRef (strict)"() -> ("Value"=w1341:refnum<vi>)  [unwired: 2 in, 2 out]
                          n322 = property on="Property Node" class="DigNum (strict)"(reference=w1341, "Value"=w1347) -> ()  [unwired: 1 in, 2 out]
                          n323 = property on="Status X" class="LVObjRef (strict)"() -> ("Value"=w1340:refnum<vi>)  [unwired: 2 in, 2 out]
                          n324 = property on="Property Node" class="Str"(reference=w1340, "Value"=w1348) -> ()  [unwired: 1 in, 2 out]
                        }
                        n325 = call "Motors Stop.vi"("error in"=w1335, "Axis"=w1326, "VISA in"=w1336) -> ("error out"=w1333:errorcluster, "VISA out"=w1334:refnum<visa-resource-name>)
                      }
                    }
                  }
                  frame #1 {
                    n326 = property on="Property Node" class="Bool (strict)"(reference=w1358, "Value"=FALSE) -> ()  [unwired: 1 in, 2 out]
                    n327 = property on="Property Node" class="Bool (strict)"(reference=w1359, "Value"=FALSE) -> ()  [unwired: 1 in, 2 out]
                  }
                }
              }
            }
            n328 = property on="y+?" class="LVObjRef (strict)"() -> ("Value"=w157:refnum<vi>)  [unwired: 2 in, 2 out]
            n329 = property on="y-?" class="LVObjRef (strict)"() -> ("Value"=w156:refnum<vi>)  [unwired: 2 in, 2 out]
            n330 = property on="Property Node" class="Bool (strict)"(reference=w157) -> (reference out=w201:refnum<vi>, "Value"=w275:bool)  [unwired: 1 in, 1 out]
            n331 = property on="Property Node" class="Bool (strict)"(reference=w156) -> (reference out=w200:refnum<vi>, "Value"=w274:bool)  [unwired: 1 in, 1 out]
            n332 = property on="Jog-Mode" class="LVObjRef (strict)"() -> ("Value"=w158:refnum<vi>)  [unwired: 2 in, 2 out]
            n333 = property on="Property Node" class="Bool (strict)"(reference=w158) -> ("Value"=w202:bool)  [unwired: 1 in, 2 out]
            n334 = Or(x=w275, y=w274) -> (x .or. y?=w301:bool)
            n335 = case shown="True" w301 {
              tunnel: w303 -> [w1188 w1197]
              tunnel: w302 -> [w1187 w1196]
              tunnel: w202 -> [_ w1198]
              tunnel: [w1188 w1195] -> w300
              tunnel: [w1187 w1194] -> w299
              tunnel: w274 -> [_ w1193]
              tunnel: w201 -> [_ w1190]
              tunnel: w200 -> [_ w1189]
              frame False {
              }
              frame True {
                n336 = flat-sequence {
                  tunnel: w1198 -> [w1205]
                  tunnel: w1197 -> [w1204]
                  tunnel: w1196 -> [w1203]
                  tunnel: w1193 -> [w1200]
                  tunnel: [w1202] -> w1192
                  tunnel: [w1201] -> w1191
                  tunnel: [w1273] -> w1194
                  tunnel: [w1274] -> w1195
                  tunnel: w1192 -> [w1274]
                  tunnel: w1191 -> [w1273]
                  tunnel: w1190 -> [w1270]
                  tunnel: w1189 -> [w1269]
                  frame #0 {
                    n337 = property on="Y Multiplier" class="LVObjRef (strict)"() -> ("Value"=w1199:refnum<vi>)  [unwired: 2 in, 2 out]
                    n338 = case shown="True" w1205 {
                      tunnel: w1204 -> [w1214 w1240]
                      tunnel: w1203 -> [w1213 w1243]
                      tunnel: [w1212 w1246] -> w1202
                      tunnel: [w1211 w1245] -> w1201
                      tunnel: w1200 -> [w1210 w1244]
                      tunnel: w1199 -> [w1208 w1235]
                      frame False {
                        n339 = property on="Y Moving" class="LVObjRef (strict)"() -> ("Value"=w1206:refnum<vi>)  [unwired: 2 in, 2 out]
                        n340 = property on="Property Node" class="Bool (strict)"(reference=w1206) -> (reference out=w1207:refnum<vi>, "Value"=w1209:bool)  [unwired: 1 in, 1 out]
                        n341 = case shown="False" w1209 {
                          tunnel: w1214 -> [w1223 w1233]
                          tunnel: w1213 -> [w1227 w1232]
                          tunnel: [w1224 w1233] -> w1212
                          tunnel: [w1226 w1232] -> w1211
                          tunnel: w1210 -> [w1225 _]
                          tunnel: w1208 -> [w1218 _]
                          tunnel: w1207 -> [w1217 _]
                          frame False {
                            n342 = property on="Delta Y (mm)" class="LVObjRef (strict)"() -> ("Value"=w1215:refnum<vi>)  [unwired: 2 in, 2 out]
                            n343 = property on="Property Node" class="DigNum (strict)"(reference=w1215) -> ("Value"=w1216:dbl)  [unwired: 1 in, 2 out]
                            n344 = property on="Property Node" class="Bool (strict)"(reference=w1217, "Value"=TRUE ("Y Moving")) -> ()  [unwired: 1 in, 2 out]
                            n345 = property on="Property Node" class="DigNum (strict)"(reference=w1218) -> ("Value"=w1220:u32)  [unwired: 1 in, 2 out]
                            n346 = case shown="True" w1225 {
                              tunnel: w1216 -> [w1228 w1230]
                              tunnel: [w1228 w1229] -> w1222
                              frame False {
                              }
                              frame True {
                                n347 = Multiply(x=w1230, y=-1.0) -> (x*y=w1229:dbl)
                              }
                            }
                            n348 = call "Motors Move Relative.vi"("Axis Multiplier"=w1220, "Axis"=2, "error in"=w1227, "VISA in"=w1223, "Distance (mm)"=w1222) -> ("error out"=w1226:errorcluster, "VISA out"=w1224:refnum<visa-resource-name>)  [unwired: 5 in]
                          }
                          frame True {
                          }
                        }
                      }
                      frame True {
                        w1237 = 2 ("Axis")
                        n349 = property on="Property Node" class="DigNum (strict)"(reference=w1235) -> ("Value"=w1238:u32)  [unwired: 1 in, 2 out]
                        n350 = property on="Y Speed (mm/s)" class="LVObjRef (strict)"() -> ("Value"=w1234:refnum<vi>)  [unwired: 2 in, 2 out]
                        n351 = property on="Property Node" class="DigNum (strict)"(reference=w1234) -> ("Value"=w1236:dbl)  [unwired: 1 in, 2 out]
                        n352 = case shown="True" w1244 {
                          tunnel: w1236 -> [w1265 w1267]
                          tunnel: [w1265 w1266] -> w1241
                          frame False {
                          }
                          frame True {
                            n353 = Multiply(x=w1267, y=-1.0) -> (x*y=w1266:dbl)
                          }
                        }
                        n354 = call "Motors Move Constant Velocity.vi"("Axis Multiplier"=w1238, "Axis"=w1237, "error in"=w1243, "VISA in"=w1240, "Speed (mm/s)"=w1241) -> ("error out"=w1242:errorcluster, "VISA out"=w1239:refnum<visa-resource-name>)  [unwired: 5 in]
                        n355 = while {
                          tunnel: w1239 -> [w1255]
                          tunnel: [w1254] -> w1248
                          tunnel: w1242 -> [w1257]
                          tunnel: [w1256] -> w1247
                          tunnel: w1238 -> [w1253]
                          stop <- w1264 continue-if-true
                          n356 = property on="y+" class="LVObjRef (strict)"() -> ("Value"=w1249:refnum<vi>)  [unwired: 2 in, 2 out]
                          n357 = property on="y-" class="LVObjRef (strict)"() -> ("Value"=w1250:refnum<vi>)  [unwired: 2 in, 2 out]
                          n358 = property on="Property Node" class="Bool (strict)"(reference=w1249) -> ("Value"=w1263:bool)  [unwired: 1 in, 2 out]
                          n359 = property on="Property Node" class="Bool (strict)"(reference=w1250) -> ("Value"=w1262:bool)  [unwired: 1 in, 2 out]
                          n360 = call "Motors Status.vi"("error in"=w1257, "VISA in"=w1255, "Axis"=2, "Axis Multiplier"=w1253) -> ("error out"=w1256:errorcluster, "VISA out"=w1254:refnum<visa-resource-name>, "OS"=w1259:i32, "Actual Position (mm or deg)"=w1260:dbl)  [unwired: 3 in]
                          n361 = Or(x=w1263, y=w1262) -> (x .or. y?=w1264:bool)
                          n362 = call "Motors Decipher Status.vi"("OS"=w1259) -> ("Status"=w1258:string)
                          n363 = property on="Y-Axis (mm)" class="LVObjRef (strict)"() -> ("Value"=w1252:refnum<vi>)  [unwired: 2 in, 2 out]
                          n364 = property on="Status Y" class="LVObjRef (strict)"() -> ("Value"=w1251:refnum<vi>)  [unwired: 2 in, 2 out]
                          n365 = property on="Property Node" class="Str"(reference=w1251, "Value"=w1258) -> ()  [unwired: 1 in, 2 out]
                          n366 = property on="Property Node" class="DigNum (strict)"(reference=w1252, "Value"=w1260) -> ()  [unwired: 1 in, 2 out]
                        }
                        n367 = call "Motors Stop.vi"("error in"=w1247, "Axis"=w1237, "VISA in"=w1248) -> ("error out"=w1245:errorcluster, "VISA out"=w1246:refnum<visa-resource-name>)
                      }
                    }
                  }
                  frame #1 {
                    n368 = property on="Property Node" class="Bool (strict)"(reference=w1270, "Value"=FALSE) -> ()  [unwired: 1 in, 2 out]
                    n369 = property on="Property Node" class="Bool (strict)"(reference=w1269, "Value"=FALSE) -> ()  [unwired: 1 in, 2 out]
                  }
                }
              }
            }
            n370 = property on="z-?" class="LVObjRef (strict)"() -> ("Value"=w153:refnum<vi>)  [unwired: 2 in, 2 out]
            n371 = property on="z+?" class="LVObjRef (strict)"() -> ("Value"=w154:refnum<vi>)  [unwired: 2 in, 2 out]
            n372 = property on="Property Node" class="Bool (strict)"(reference=w153) -> (reference out=w242:refnum<vi>, "Value"=w273:bool)  [unwired: 1 in, 1 out]
            n373 = property on="Property Node" class="Bool (strict)"(reference=w154) -> (reference out=w241:refnum<vi>, "Value"=w272:bool)  [unwired: 1 in, 1 out]
            n374 = property on="Jog-Mode" class="LVObjRef (strict)"() -> ("Value"=w155:refnum<vi>)  [unwired: 2 in, 2 out]
            n375 = property on="Property Node" class="Bool (strict)"(reference=w155) -> ("Value"=w199:bool)  [unwired: 1 in, 2 out]
            n376 = Or(x=w272, y=w273) -> (x .or. y?=w298:bool)
            n377 = case shown="True" w298 {
              tunnel: w300 -> [w1096 w1106]
              tunnel: w299 -> [w1095 w1100]
              tunnel: w199 -> [_ w1107]
              tunnel: [w1096 w1105] -> w295
              tunnel: [w1095 w1104] -> w296
              tunnel: w273 -> [_ w1103]
              tunnel: w242 -> [_ w1099]
              tunnel: w242 -> [_ w1098]
              tunnel: w241 -> [_ w1097]
              frame False {
              }
              frame True {
                n378 = flat-sequence {
                  tunnel: w1107 -> [w1115]
                  tunnel: w1106 -> [w1114]
                  tunnel: w1103 -> [w1111]
                  tunnel: [w1113] -> w1102
                  tunnel: [w1112] -> w1101
                  tunnel: w1100 -> [w1110]
                  tunnel: w1099 -> [w1109]
                  tunnel: [w1185] -> w1104
                  tunnel: [w1186] -> w1105
                  tunnel: w1102 -> [w1186]
                  tunnel: w1101 -> [w1185]
                  tunnel: w1098 -> [w1182]
                  tunnel: w1097 -> [w1181]
                  frame #0 {
                    n379 = property on="Z Multiplier" class="LVObjRef (strict)"() -> ("Value"=w1108:refnum<vi>)  [unwired: 2 in, 2 out]
                    n380 = case shown="False" w1115 {
                      tunnel: w1114 -> [w1124 w1152]
                      tunnel: w1110 -> [w1123 w1155]
                      tunnel: [w1122 w1158] -> w1113
                      tunnel: [w1121 w1157] -> w1112
                      tunnel: w1111 -> [w1120 w1147]
                      tunnel: w1110 -> [_ w1149]
                      tunnel: w1109 -> [_ w1146]
                      tunnel: w1108 -> [w1117 w1145]
                      frame False {
                        n381 = property on="Z Moving" class="LVObjRef (strict)"() -> ("Value"=w1116:refnum<vi>)  [unwired: 2 in, 2 out]
                        n382 = property on="Property Node" class="Bool (strict)"(reference=w1116) -> (reference out=w1118:refnum<vi>, "Value"=w1119:bool)  [unwired: 1 in, 1 out]
                        n383 = case shown="False" w1119 {
                          tunnel: w1124 -> [w1130 w1143]
                          tunnel: w1123 -> [w1137 w1142]
                          tunnel: [w1131 w1143] -> w1122
                          tunnel: [w1136 w1142] -> w1121
                          tunnel: w1120 -> [w1135 _]
                          tunnel: w1118 -> [w1127 _]
                          tunnel: w1117 -> [w1126 _]
                          frame False {
                            n384 = property on="Delta Z (mm)" class="LVObjRef (strict)"() -> ("Value"=w1125:refnum<vi>)  [unwired: 2 in, 2 out]
                            n385 = property on="Property Node" class="DigNum (strict)"(reference=w1125) -> ("Value"=w1128:dbl)  [unwired: 1 in, 2 out]
                            n386 = property on="Property Node" class="Bool (strict)"(reference=w1127, "Value"=TRUE ("Z Moving")) -> ()  [unwired: 1 in, 2 out]
                            n387 = property on="Property Node" class="DigNum (strict)"(reference=w1126) -> ("Value"=w1133:u32)  [unwired: 1 in, 2 out]
                            n388 = case shown="True" w1135 {
                              tunnel: w1128 -> [w1138 w1140]
                              tunnel: [w1138 w1139] -> w1132
                              frame False {
                              }
                              frame True {
                                n389 = Multiply(x=w1140, y=-1.0) -> (x*y=w1139:dbl)
                              }
                            }
                            n390 = call "Motors Move Relative.vi"("Axis Multiplier"=w1133, "Axis"=3, "error in"=w1137, "VISA in"=w1130, "Distance (mm)"=w1132) -> ("error out"=w1136:errorcluster, "VISA out"=w1131:refnum<visa-resource-name>)  [unwired: 5 in]
                          }
                          frame True {
                          }
                        }
                      }
                      frame True {
                        w1154 = 3 ("Axis")
                        n391 = property on="Property Node" class="DigNum (strict)"(reference=w1145) -> ("Value"=w1150:u32)  [unwired: 1 in, 2 out]
                        n392 = property on="Z Speed (mm/s)" class="LVObjRef (strict)"() -> ("Value"=w1144:refnum<vi>)  [unwired: 2 in, 2 out]
                        n393 = property on="Property Node" class="DigNum (strict)"(reference=w1144, error in=w1149) -> ("Value"=w1148:dbl)  [unwired: 2 out]
                        n394 = case shown="True" w1147 {
                          tunnel: w1148 -> [w1177 w1179]
                          tunnel: [w1177 w1178] -> w1153
                          frame False {
                          }
                          frame True {
                            n395 = Multiply(x=w1179, y=-1.0) -> (x*y=w1178:dbl)
                          }
                        }
                        n396 = call "Motors Move Constant Velocity.vi"("Axis Multiplier"=w1150, "Axis"=w1154, "error in"=w1155, "VISA in"=w1152, "Speed (mm/s)"=w1153) -> ("error out"=w1156:errorcluster, "VISA out"=w1151:refnum<visa-resource-name>)  [unwired: 5 in]
                        n397 = while {
                          tunnel: w1151 -> [w1167]
                          tunnel: [w1166] -> w1160
                          tunnel: w1156 -> [w1169]
                          tunnel: [w1168] -> w1159
                          tunnel: w1150 -> [w1165]
                          tunnel: w1146 -> [_]
                          stop <- w1176 continue-if-true
                          n398 = property on="z+" class="LVObjRef (strict)"() -> ("Value"=w1163:refnum<vi>)  [unwired: 2 in, 2 out]
                          n399 = property on="z-" class="LVObjRef (strict)"() -> ("Value"=w1162:refnum<vi>)  [unwired: 2 in, 2 out]
                          n400 = property on="Property Node" class="Bool (strict)"(reference=w1163) -> ("Value"=w1175:bool)  [unwired: 1 in, 2 out]
                          n401 = property on="Property Node" class="Bool (strict)"(reference=w1162) -> ("Value"=w1174:bool)  [unwired: 1 in, 2 out]
                          n402 = call "Motors Status.vi"("error in"=w1169, "VISA in"=w1167, "Axis"=3, "Axis Multiplier"=w1165) -> ("error out"=w1168:errorcluster, "VISA out"=w1166:refnum<visa-resource-name>, "OS"=w1171:i32, "Actual Position (mm or deg)"=w1172:dbl)  [unwired: 3 in]
                          n403 = Or(x=w1175, y=w1174) -> (x .or. y?=w1176:bool)
                          n404 = call "Motors Decipher Status.vi"("OS"=w1171) -> ("Status"=w1170:string)
                          n405 = property on="Z-Axis (mm)" class="LVObjRef (strict)"() -> ("Value"=w1161:refnum<vi>)  [unwired: 2 in, 2 out]
                          n406 = property on="Status Z" class="LVObjRef (strict)"() -> ("Value"=w1164:refnum<vi>)  [unwired: 2 in, 2 out]
                          n407 = property on="Property Node" class="Str"(reference=w1164, "Value"=w1170) -> ()  [unwired: 1 in, 2 out]
                          n408 = property on="Property Node" class="DigNum (strict)"(reference=w1161, "Value"=w1172) -> ()  [unwired: 1 in, 2 out]
                        }
                        n409 = call "Motors Stop.vi"("error in"=w1159, "Axis"=w1154, "VISA in"=w1160) -> ("error out"=w1157:errorcluster, "VISA out"=w1158:refnum<visa-resource-name>)
                      }
                    }
                  }
                  frame #1 {
                    n410 = property on="Property Node" class="Bool (strict)"(reference=w1182, "Value"=FALSE) -> ()  [unwired: 1 in, 2 out]
                    n411 = property on="Property Node" class="Bool (strict)"(reference=w1181, "Value"=FALSE) -> ()  [unwired: 1 in, 2 out]
                  }
                }
              }
            }
            n412 = property on="theta-?" class="LVObjRef (strict)"() -> ("Value"=w150:refnum<vi>)  [unwired: 2 in, 2 out]
            n413 = property on="theta+?" class="LVObjRef (strict)"() -> ("Value"=w151:refnum<vi>)  [unwired: 2 in, 2 out]
            n414 = property on="Property Node" class="Bool (strict)"(reference=w151) -> (reference out=w197:refnum<vi>, "Value"=w271:bool)  [unwired: 1 in, 1 out]
            n415 = property on="Property Node" class="Bool (strict)"(reference=w150) -> (reference out=w198:refnum<vi>, "Value"=w270:bool)  [unwired: 1 in, 1 out]
            n416 = property on="Jog-Mode" class="LVObjRef (strict)"() -> ("Value"=w152:refnum<vi>)  [unwired: 2 in, 2 out]
            n417 = property on="Property Node" class="Bool (strict)"(reference=w152) -> ("Value"=w204:bool)  [unwired: 1 in, 2 out]
            n418 = Or(x=w271, y=w270) -> (x .or. y?=w297:bool)
            n419 = case shown="True" w297 {
              tunnel: w295 -> [w1008 w1017]
              tunnel: w296 -> [w1007 w1016]
              tunnel: w204 -> [_ w1018]
              tunnel: [w1008 w1015] -> w294
              tunnel: [w1007 w1014] -> w287
              tunnel: w270 -> [_ w1013]
              tunnel: w198 -> [_ w1010]
              tunnel: w197 -> [_ w1009]
              frame False {
              }
              frame True {
                n420 = flat-sequence {
                  tunnel: w1018 -> [w1025]
                  tunnel: w1017 -> [w1024]
                  tunnel: w1016 -> [w1023]
                  tunnel: w1013 -> [w1020]
                  tunnel: [w1022] -> w1012
                  tunnel: [w1021] -> w1011
                  tunnel: [w1093] -> w1014
                  tunnel: [w1094] -> w1015
                  tunnel: w1012 -> [w1094]
                  tunnel: w1011 -> [w1093]
                  tunnel: w1010 -> [w1090]
                  tunnel: w1009 -> [w1089]
                  frame #0 {
                    n421 = property on="Theta Multiplier" class="LVObjRef (strict)"() -> ("Value"=w1019:refnum<vi>)  [unwired: 2 in, 2 out]
                    n422 = case shown="True" w1025 {
                      tunnel: w1024 -> [w1034 w1061]
                      tunnel: w1023 -> [w1033 w1062]
                      tunnel: [w1032 w1066] -> w1022
                      tunnel: [w1031 w1065] -> w1021
                      tunnel: w1020 -> [w1030 w1064]
                      tunnel: w1019 -> [w1028 w1056]
                      frame False {
                        n423 = property on="Theta Moving" class="LVObjRef (strict)"() -> ("Value"=w1026:refnum<vi>)  [unwired: 2 in, 2 out]
                        n424 = property on="Property Node" class="Bool (strict)"(reference=w1026) -> (reference out=w1027:refnum<vi>, "Value"=w1029:bool)  [unwired: 1 in, 1 out]
                        n425 = case shown="False" w1029 {
                          tunnel: w1034 -> [w1041 w1053]
                          tunnel: w1033 -> [w1047 w1052]
                          tunnel: [w1042 w1053] -> w1032
                          tunnel: [w1046 w1052] -> w1031
                          tunnel: w1030 -> [w1045 _]
                          tunnel: w1028 -> [w1038 _]
                          tunnel: w1027 -> [w1037 _]
                          frame False {
                            n426 = property on="Delta Theta (deg)" class="LVObjRef (strict)"() -> ("Value"=w1035:refnum<vi>)  [unwired: 2 in, 2 out]
                            n427 = property on="Property Node" class="DigNum (strict)"(reference=w1035) -> ("Value"=w1036:dbl)  [unwired: 1 in, 2 out]
                            n428 = property on="Property Node" class="Bool (strict)"(reference=w1037, "Value"=TRUE ("Theta Moving")) -> ()  [unwired: 1 in, 2 out]
                            n429 = property on="Property Node" class="DigNum (strict)"(reference=w1038) -> ("Value"=w1044:u32)  [unwired: 1 in, 2 out]
                            n430 = case shown="True" w1045 {
                              tunnel: w1036 -> [w1048 w1050]
                              tunnel: [w1048 w1049] -> w1040
                              frame False {
                              }
                              frame True {
                                n431 = Multiply(x=w1050, y=-1.0) -> (x*y=w1049:dbl)
                              }
                            }
                            n432 = call "Motors Move Relative.vi"("Axis Multiplier"=w1044, "Axis"=4, "error in"=w1047, "VISA in"=w1041, "Distance (mm)"=w1040) -> ("error out"=w1046:errorcluster, "VISA out"=w1042:refnum<visa-resource-name>)  [unwired: 5 in]
                          }
                          frame True {
                          }
                        }
                      }
                      frame True {
                        w1059 = 4 ("Axis")
                        n433 = property on="Property Node" class="DigNum (strict)"(reference=w1056) -> ("Value"=w1058:u32)  [unwired: 1 in, 2 out]
                        n434 = property on="Theta Speed (deg/s)" class="LVObjRef (strict)"() -> ("Value"=w1054:refnum<vi>)  [unwired: 2 in, 2 out]
                        n435 = property on="Property Node" class="DigNum (strict)"(reference=w1054) -> ("Value"=w1055:dbl)  [unwired: 1 in, 2 out]
                        n436 = case shown="True" w1064 {
                          tunnel: w1055 -> [w1085 w1087]
                          tunnel: [w1085 w1086] -> w1057
                          frame False {
                          }
                          frame True {
                            n437 = Multiply(x=w1087, y=-1.0) -> (x*y=w1086:dbl)
                          }
                        }
                        n438 = call "Motors Move Constant Velocity.vi"("Axis Multiplier"=w1058, "Axis"=w1059, "error in"=w1062, "VISA in"=w1061, "Speed (mm/s)"=w1057) -> ("error out"=w1063:errorcluster, "VISA out"=w1060:refnum<visa-resource-name>)  [unwired: 5 in]
                        n439 = while {
                          tunnel: w1060 -> [w1075]
                          tunnel: [w1074] -> w1068
                          tunnel: w1063 -> [w1077]
                          tunnel: [w1076] -> w1067
                          tunnel: w1058 -> [w1073]
                          stop <- w1084 continue-if-true
                          n440 = property on="theta+" class="LVObjRef (strict)"() -> ("Value"=w1070:refnum<vi>)  [unwired: 2 in, 2 out]
                          n441 = property on="theta-" class="LVObjRef (strict)"() -> ("Value"=w1071:refnum<vi>)  [unwired: 2 in, 2 out]
                          n442 = property on="Property Node" class="Bool (strict)"(reference=w1070) -> ("Value"=w1083:bool)  [unwired: 1 in, 2 out]
                          n443 = property on="Property Node" class="Bool (strict)"(reference=w1071) -> ("Value"=w1082:bool)  [unwired: 1 in, 2 out]
                          n444 = call "Motors Status.vi"("error in"=w1077, "VISA in"=w1075, "Axis"=4, "Axis Multiplier"=w1073) -> ("error out"=w1076:errorcluster, "VISA out"=w1074:refnum<visa-resource-name>, "OS"=w1079:i32, "Actual Position (mm or deg)"=w1080:dbl)  [unwired: 3 in]
                          n445 = Or(x=w1083, y=w1082) -> (x .or. y?=w1084:bool)
                          n446 = call "Motors Decipher Status.vi"("OS"=w1079) -> ("Status"=w1078:string)
                          n447 = property on="Theta (deg)" class="LVObjRef (strict)"() -> ("Value"=w1069:refnum<vi>)  [unwired: 2 in, 2 out]
                          n448 = property on="Status Theta" class="LVObjRef (strict)"() -> ("Value"=w1072:refnum<vi>)  [unwired: 2 in, 2 out]
                          n449 = property on="Property Node" class="Str"(reference=w1072, "Value"=w1078) -> ()  [unwired: 1 in, 2 out]
                          n450 = property on="Property Node" class="DigNum (strict)"(reference=w1069, "Value"=w1080) -> ()  [unwired: 1 in, 2 out]
                        }
                        n451 = call "Motors Stop.vi"("error in"=w1067, "Axis"=w1059, "VISA in"=w1068) -> ("error out"=w1065:errorcluster, "VISA out"=w1066:refnum<visa-resource-name>)
                      }
                    }
                  }
                  frame #1 {
                    n452 = property on="Property Node" class="Bool (strict)"(reference=w1089, "Value"=FALSE) -> ()  [unwired: 1 in, 2 out]
                    n453 = property on="Property Node" class="Bool (strict)"(reference=w1090, "Value"=FALSE) -> ()  [unwired: 1 in, 2 out]
                  }
                }
              }
            }
            n454 = property on="X Set Slew Speed?" class="LVObjRef (strict)"() -> ("Value"=w174:refnum<vi>)  [unwired: 2 in, 2 out]
            n455 = property on="Property Node" class="Bool (strict)"(reference=w174) -> (reference out=w192:refnum<vi>, "Value"=w196:bool)  [unwired: 1 in, 1 out]
            n456 = case shown="True" w196 {
              tunnel: [w993 w1001] -> w291
              tunnel: w294 -> [w993 w1002]
              tunnel: [w992 w1005] -> w288
              tunnel: w287 -> [w992 w1006]
              tunnel: w192 -> [_ w997]
              frame False {
              }
              frame True {
                n457 = property on="(mm/s)" class="LVObjRef (strict)"() -> ("Value"=w995:refnum<vi>)  [unwired: 2 in, 2 out]
                n458 = property on="Need to Update Motor Parameters" class="LVObjRef (strict)"() -> ("Value"=w994:refnum<vi>)  [unwired: 2 in, 2 out]
                n459 = property on="X Multiplier" class="LVObjRef (strict)"() -> ("Value"=w996:refnum<vi>)  [unwired: 2 in, 2 out]
                n460 = property on="Property Node" class="DigNum (strict)"(reference=w995) -> ("Value"=w999:dbl)  [unwired: 1 in, 2 out]
                n461 = property on="Property Node" class="DigNum (strict)"(reference=w996) -> ("Value"=w1000:u32)  [unwired: 1 in, 2 out]
                n462 = property on="Property Node" class="Bool (strict)"(reference=w997, "Value"=FALSE) -> ()  [unwired: 1 in, 2 out]
                n463 = property on="Property Node" class="Bool (strict)"(reference=w994, "Value"=TRUE ("Need to Update Motor Parameters")) -> ()  [unwired: 1 in, 2 out]
                n464 = call "Motors Move Speed.vi"("Speed (mm or degree/sec)"=w999, "error in"=w1006, "VISA in"=w1002, "Axis"=u32 1, "Axis Multiplier"=w1000) -> ("error out"=w1005:errorcluster, "VISA out"=w1001:refnum<visa-resource-name>)  [unwired: 5 in]
              }
            }
            n465 = property on="Y Set Slew Speed?" class="LVObjRef (strict)"() -> ("Value"=w173:refnum<vi>)  [unwired: 2 in, 2 out]
            n466 = property on="Property Node" class="Bool (strict)"(reference=w173) -> (reference out=w191:refnum<vi>, "Value"=w195:bool)  [unwired: 1 in, 1 out]
            n467 = case shown="True" w195 {
              tunnel: [w978 w987] -> w292
              tunnel: w291 -> [w978 w985]
              tunnel: [w977 w990] -> w289
              tunnel: w288 -> [w977 w991]
              tunnel: w191 -> [_ w982]
              frame False {
              }
              frame True {
                n468 = property on="Need to Update Motor Parameters" class="LVObjRef (strict)"() -> ("Value"=w979:refnum<vi>)  [unwired: 2 in, 2 out]
                n469 = property on="(mm/s) 2" class="LVObjRef (strict)"() -> ("Value"=w980:refnum<vi>)  [unwired: 2 in, 2 out]
                n470 = property on="Y Multiplier" class="LVObjRef (strict)"() -> ("Value"=w981:refnum<vi>)  [unwired: 2 in, 2 out]
                n471 = property on="Property Node" class="DigNum (strict)"(reference=w980) -> ("Value"=w984:dbl)  [unwired: 1 in, 2 out]
                n472 = property on="Property Node" class="DigNum (strict)"(reference=w981) -> ("Value"=w986:u32)  [unwired: 1 in, 2 out]
                n473 = property on="Property Node" class="Bool (strict)"(reference=w982, "Value"=FALSE) -> ()  [unwired: 1 in, 2 out]
                n474 = property on="Property Node" class="Bool (strict)"(reference=w979, "Value"=TRUE ("Need to Update Motor Parameters")) -> ()  [unwired: 1 in, 2 out]
                n475 = call "Motors Move Speed.vi"("Speed (mm or degree/sec)"=w984, "error in"=w991, "VISA in"=w985, "Axis"=u32 2, "Axis Multiplier"=w986) -> ("error out"=w990:errorcluster, "VISA out"=w987:refnum<visa-resource-name>)  [unwired: 5 in]
              }
            }
            n476 = property on="Z Set Slew Speed?" class="LVObjRef (strict)"() -> ("Value"=w172:refnum<vi>)  [unwired: 2 in, 2 out]
            n477 = property on="Property Node" class="Bool (strict)"(reference=w172) -> (reference out=w190:refnum<vi>, "Value"=w194:bool)  [unwired: 1 in, 1 out]
            n478 = case shown="True" w194 {
              tunnel: [w963 w972] -> w293
              tunnel: w292 -> [w963 w971]
              tunnel: [w962 w975] -> w290
              tunnel: w289 -> [w962 w976]
              tunnel: w190 -> [_ w967]
              frame False {
              }
              frame True {
                n479 = property on="Need to Update Motor Parameters" class="LVObjRef (strict)"() -> ("Value"=w964:refnum<vi>)  [unwired: 2 in, 2 out]
                n480 = property on="(mm/s) 3" class="LVObjRef (strict)"() -> ("Value"=w965:refnum<vi>)  [unwired: 2 in, 2 out]
                n481 = property on="Z Multiplier" class="LVObjRef (strict)"() -> ("Value"=w966:refnum<vi>)  [unwired: 2 in, 2 out]
                n482 = property on="Property Node" class="DigNum (strict)"(reference=w965) -> ("Value"=w969:dbl)  [unwired: 1 in, 2 out]
                n483 = property on="Property Node" class="DigNum (strict)"(reference=w966) -> ("Value"=w970:u32)  [unwired: 1 in, 2 out]
                n484 = property on="Property Node" class="Bool (strict)"(reference=w967, "Value"=FALSE) -> ()  [unwired: 1 in, 2 out]
                n485 = property on="Property Node" class="Bool (strict)"(reference=w964, "Value"=TRUE ("Need to Update Motor Parameters")) -> ()  [unwired: 1 in, 2 out]
                n486 = call "Motors Move Speed.vi"("Speed (mm or degree/sec)"=w969, "error in"=w976, "VISA in"=w971, "Axis"=u32 3, "Axis Multiplier"=w970) -> ("error out"=w975:errorcluster, "VISA out"=w972:refnum<visa-resource-name>)  [unwired: 5 in]
              }
            }
            n487 = property on="Theta Set Slew Speed?" class="LVObjRef (strict)"() -> ("Value"=w171:refnum<vi>)  [unwired: 2 in, 2 out]
            n488 = property on="Property Node" class="Bool (strict)"(reference=w171) -> (reference out=w189:refnum<vi>, "Value"=w193:bool)  [unwired: 1 in, 1 out]
            n489 = case shown="True" w193 {
              tunnel: [w948 w957] -> w285
              tunnel: w293 -> [w948 w956]
              tunnel: [w947 w958] -> w286
              tunnel: w290 -> [w947 w961]
              tunnel: w189 -> [_ w952]
              frame False {
              }
              frame True {
                n490 = property on="Theta Multiplier" class="LVObjRef (strict)"() -> ("Value"=w951:refnum<vi>)  [unwired: 2 in, 2 out]
                n491 = property on="Need to Update Motor Parameters" class="LVObjRef (strict)"() -> ("Value"=w949:refnum<vi>)  [unwired: 2 in, 2 out]
                n492 = property on="(degrees/s)" class="LVObjRef (strict)"() -> ("Value"=w950:refnum<vi>)  [unwired: 2 in, 2 out]
                n493 = property on="Property Node" class="DigNum (strict)"(reference=w950) -> ("Value"=w954:dbl)  [unwired: 1 in, 2 out]
                n494 = property on="Property Node" class="DigNum (strict)"(reference=w951) -> ("Value"=w955:u32)  [unwired: 1 in, 2 out]
                n495 = property on="Property Node" class="Bool (strict)"(reference=w952, "Value"=FALSE) -> ()  [unwired: 1 in, 2 out]
                n496 = property on="Property Node" class="Bool (strict)"(reference=w949, "Value"=TRUE ("Need to Update Motor Parameters")) -> ()  [unwired: 1 in, 2 out]
                n497 = call "Motors Move Speed.vi"("Speed (mm or degree/sec)"=w954, "error in"=w961, "VISA in"=w956, "Axis"=u32 4, "Axis Multiplier"=w955) -> ("error out"=w958:errorcluster, "VISA out"=w957:refnum<visa-resource-name>)  [unwired: 5 in]
              }
            }
            n498 = Quotient & Remainder(x=w263, y=4) -> (x-y*floor(x/y)=w283:i32)  [unwired: 1 out]
            n499 = case shown="3" w283 {
              tunnel: w286 -> [w787 w805 w822 w841]
              tunnel: w285 -> [w788 w806 w824 w842]
              tunnel: [w786 w803 w821 w840] -> w281
              tunnel: [w785 w804 w823 w839] -> w280
              frame 0, Default {
                n500 = property on="X Multiplier" class="LVObjRef (strict)"() -> ("Value"=w781:refnum<vi>)  [unwired: 2 in, 2 out]
                n501 = property on="Property Node" class="DigNum (strict)"(reference=w781) -> ("Value"=w784:u32)  [unwired: 1 in, 2 out]
                n502 = call "Motors Status.vi"("error in"=w787, "VISA in"=w788, "Axis"=1, "Axis Multiplier"=w784) -> ("error out"=w786:errorcluster, "VISA out"=w785:refnum<visa-resource-name>, "OS"=w794:i32, "Actual Position (mm or deg)"=w789:dbl)  [unwired: 3 in]
                n503 = call "Motors Decipher Status.vi"("OS"=w794) -> ("Status"=w793:string)
                n504 = Equal?(x=w793, y="Idle") -> (x = y?=w791:bool)
                n505 = case shown="False" w791 {
                  tunnel: [TRUE FALSE] -> w790
                  frame False {
                  }
                  frame True {
                  }
                }
                n506 = property on="X Moving" class="LVObjRef (strict)"() -> ("Value"=w782:refnum<vi>)  [unwired: 2 in, 2 out]
                n507 = property on="X-Axis (mm)" class="LVObjRef (strict)"() -> ("Value"=w780:refnum<vi>)  [unwired: 2 in, 2 out]
                n508 = property on="Status X" class="LVObjRef (strict)"() -> ("Value"=w783:refnum<vi>)  [unwired: 2 in, 2 out]
                n509 = property on="Property Node" class="DigNum (strict)"(reference=w780, "Value"=w789) -> ()  [unwired: 1 in, 2 out]
                n510 = property on="Property Node" class="Bool (strict)"(reference=w782, "Value"=w790) -> ()  [unwired: 1 in, 2 out]
                n511 = property on="Property Node" class="Str"(reference=w783, "Value"=w793) -> ()  [unwired: 1 in, 2 out]
              }
              frame 1 {
                n512 = property on="Y Multiplier" class="LVObjRef (strict)"() -> ("Value"=w799:refnum<vi>)  [unwired: 2 in, 2 out]
                n513 = property on="Property Node" class="DigNum (strict)"(reference=w799) -> ("Value"=w802:u32)  [unwired: 1 in, 2 out]
                n514 = call "Motors Status.vi"("error in"=w805, "VISA in"=w806, "Axis"=2, "Axis Multiplier"=w802) -> ("error out"=w803:errorcluster, "VISA out"=w804:refnum<visa-resource-name>, "OS"=w811:i32, "Actual Position (mm or deg)"=w812:dbl)  [unwired: 3 in]
                n515 = call "Motors Decipher Status.vi"("OS"=w811) -> ("Status"=w809:string)
                n516 = Equal?(x=w809, y="Idle") -> (x = y?=w808:bool)
                n517 = case shown="False" w808 {
                  tunnel: [TRUE FALSE] -> w807
                  frame False {
                  }
                  frame True {
                  }
                }
                n518 = property on="Y Moving" class="LVObjRef (strict)"() -> ("Value"=w801:refnum<vi>)  [unwired: 2 in, 2 out]
                n519 = property on="Y-Axis (mm)" class="LVObjRef (strict)"() -> ("Value"=w798:refnum<vi>)  [unwired: 2 in, 2 out]
                n520 = property on="Status Y" class="LVObjRef (strict)"() -> ("Value"=w800:refnum<vi>)  [unwired: 2 in, 2 out]
                n521 = property on="Property Node" class="DigNum (strict)"(reference=w798, "Value"=w812) -> ()  [unwired: 1 in, 2 out]
                n522 = property on="Property Node" class="Bool (strict)"(reference=w801, "Value"=w807) -> ()  [unwired: 1 in, 2 out]
                n523 = property on="Property Node" class="Str"(reference=w800, "Value"=w809) -> ()  [unwired: 1 in, 2 out]
              }
              frame 2 {
                n524 = property on="Z Multiplier" class="LVObjRef (strict)"() -> ("Value"=w818:refnum<vi>)  [unwired: 2 in, 2 out]
                n525 = property on="Property Node" class="DigNum (strict)"(reference=w818) -> ("Value"=w820:u32)  [unwired: 1 in, 2 out]
                n526 = call "Motors Status.vi"("error in"=w822, "VISA in"=w824, "Axis"=3, "Axis Multiplier"=w820) -> ("error out"=w821:errorcluster, "VISA out"=w823:refnum<visa-resource-name>, "OS"=w829:i32, "Actual Position (mm or deg)"=w830:dbl)  [unwired: 3 in]
                n527 = call "Motors Decipher Status.vi"("OS"=w829) -> ("Status"=w827:string)
                n528 = Equal?(x=w827, y="Idle") -> (x = y?=w826:bool)
                n529 = case shown="False" w826 {
                  tunnel: [TRUE FALSE] -> w825
                  frame False {
                  }
                  frame True {
                  }
                }
                n530 = property on="Z Moving" class="LVObjRef (strict)"() -> ("Value"=w817:refnum<vi>)  [unwired: 2 in, 2 out]
                n531 = property on="Z-Axis (mm)" class="LVObjRef (strict)"() -> ("Value"=w816:refnum<vi>)  [unwired: 2 in, 2 out]
                n532 = property on="Status Z" class="LVObjRef (strict)"() -> ("Value"=w819:refnum<vi>)  [unwired: 2 in, 2 out]
                n533 = property on="Property Node" class="DigNum (strict)"(reference=w816, "Value"=w830) -> ()  [unwired: 1 in, 2 out]
                n534 = property on="Property Node" class="Str"(reference=w819, "Value"=w827) -> ()  [unwired: 1 in, 2 out]
                n535 = property on="Property Node" class="Bool (strict)"(reference=w817, "Value"=w825) -> ()  [unwired: 1 in, 2 out]
              }
              frame 3 {
                n536 = property on="Theta Multiplier" class="LVObjRef (strict)"() -> ("Value"=w836:refnum<vi>)  [unwired: 2 in, 2 out]
                n537 = property on="Property Node" class="DigNum (strict)"(reference=w836) -> ("Value"=w838:u32)  [unwired: 1 in, 2 out]
                n538 = call "Motors Status.vi"("error in"=w841, "VISA in"=w842, "Axis"=4, "Axis Multiplier"=w838) -> ("error out"=w840:errorcluster, "VISA out"=w839:refnum<visa-resource-name>, "OS"=w847:i32, "Actual Position (mm or deg)"=w848:dbl)  [unwired: 3 in]
                n539 = call "Motors Decipher Status.vi"("OS"=w847) -> ("Status"=w845:string)
                n540 = Equal?(x=w845, y="Idle") -> (x = y?=w844:bool)
                n541 = case shown="True" w844 {
                  tunnel: [TRUE FALSE] -> w843
                  frame False {
                  }
                  frame True {
                  }
                }
                n542 = property on="Theta (deg)" class="LVObjRef (strict)"() -> ("Value"=w834:refnum<vi>)  [unwired: 2 in, 2 out]
                n543 = property on="Status Theta" class="LVObjRef (strict)"() -> ("Value"=w837:refnum<vi>)  [unwired: 2 in, 2 out]
                n544 = property on="Theta Moving" class="LVObjRef (strict)"() -> ("Value"=w835:refnum<vi>)  [unwired: 2 in, 2 out]
                n545 = property on="Property Node" class="DigNum (strict)"(reference=w834, "Value"=w848) -> ()  [unwired: 1 in, 2 out]
                n546 = property on="Property Node" class="Str"(reference=w837, "Value"=w845) -> ()  [unwired: 1 in, 2 out]
                n547 = property on="Property Node" class="Bool (strict)"(reference=w835, "Value"=w843) -> ()  [unwired: 1 in, 2 out]
              }
            }
            n548 = property on="Go To Saved Position?" class="LVObjRef (strict)"() -> ("Value"=w149:refnum<vi>)  [unwired: 2 in, 2 out]
            n549 = property on="Property Node" class="Bool (strict)"(reference=w149) -> (reference out=w187:refnum<vi>, "Value"=w188:bool)  [unwired: 1 in, 1 out]
            n550 = case shown="True" w188 {
              tunnel: w281 -> [w741 w752]
              tunnel: w280 -> [w740 w758]
              tunnel: [w741 w771] -> w279
              tunnel: [w740 w770] -> w278
              tunnel: w187 -> [_ w749]
              frame False {
              }
              frame True {
                w768 = 4 ("index (row)")
                w766 = 3 ("index (row)")
                w763 = 2 ("index (row)")
                w760 = 1 ("index (row)")
                n551 = property on="Property Node" class="Bool (strict)"(reference=w749, "Value"=FALSE) -> ()  [unwired: 1 in, 2 out]
                n552 = property on="Theta Multiplier" class="LVObjRef (strict)"() -> ("Value"=w744:refnum<vi>)  [unwired: 2 in, 2 out]
                n553 = property on="Defined Positions" class="LVObjRef (strict)"() -> ("Value"=w742:refnum<vi>)  [unwired: 2 in, 2 out]
                n554 = property on="Saved Positions" class="LVObjRef (strict)"() -> ("Value"=w743:refnum<vi>)  [unwired: 2 in, 2 out]
                n555 = property on="Z Multiplier" class="LVObjRef (strict)"() -> ("Value"=w745:refnum<vi>)  [unwired: 2 in, 2 out]
                n556 = property on="Y Multiplier" class="LVObjRef (strict)"() -> ("Value"=w746:refnum<vi>)  [unwired: 2 in, 2 out]
                n557 = property on="X Multiplier" class="LVObjRef (strict)"() -> ("Value"=w747:refnum<vi>)  [unwired: 2 in, 2 out]
                n558 = property on="Property Node" class="DigNum (strict)"(reference=w744) -> ("Value"=w754:u32)  [unwired: 1 in, 2 out]
                n559 = property on="Property Node" class="DigNum (strict)"(reference=w745) -> ("Value"=w755:u32)  [unwired: 1 in, 2 out]
                n560 = property on="Property Node" class="DigNum (strict)"(reference=w746) -> ("Value"=w756:u32)  [unwired: 1 in, 2 out]
                n561 = property on="Property Node" class="DigNum (strict)"(reference=w747) -> ("Value"=w757:u32)  [unwired: 1 in, 2 out]
                n562 = property on="Property Node" class="Path"(reference=w743) -> ("Value"=w753:path)  [unwired: 1 in, 2 out]
                n563 = property on="Property Node" class="LstBox (strict)"(reference=w742) -> ("Value"=w748:i32)  [unwired: 1 in, 2 out]
                n564 = call "Motors Position Load.vi"("error in"=w752, "file path"=w753) -> ("error out"=w751:errorcluster, "Positions"=w774:string[][])
                n565 = Index Array(array=w774, index (row)=w768, index (col)=w748) -> (element=w775:string)
                n566 = Index Array(array=w774, index (row)=w766, index (col)=w748) -> (element=w776:string)
                n567 = Index Array(array=w774, index (row)=w763, index (col)=w748) -> (element=w778:string)
                n568 = Index Array(array=w774, index (row)=w760, index (col)=w748) -> (element=w779:string)
                n569 = Fract/Exp String To Number(string=w775) -> (number=w769:dbl)  [unwired: 3 in, 1 out]
                n570 = Fract/Exp String To Number(string=w776) -> (number=w765:dbl)  [unwired: 3 in, 1 out]
                n571 = Fract/Exp String To Number(string=w778) -> (number=w762:dbl)  [unwired: 3 in, 1 out]
                n572 = Fract/Exp String To Number(string=w779) -> (number=w759:dbl)  [unwired: 3 in, 1 out]
                n573 = call "Motors Move Absolute.vi"("Axis Multiplier"=w757, "Axis"=w760, "error in"=w751, "VISA in"=w758, "Position (mm or degree)"=w759) -> ("error out"=w777:errorcluster, "VISA out"=w761:refnum<visa-resource-name>)  [unwired: 5 in]
                n574 = call "Motors Move Absolute.vi"("Axis Multiplier"=w756, "Axis"=w763, "error in"=w777, "VISA in"=w761, "Position (mm or degree)"=w762) -> ("error out"=w773:errorcluster, "VISA out"=w764:refnum<visa-resource-name>)  [unwired: 5 in]
                n575 = call "Motors Move Absolute.vi"("Axis Multiplier"=w755, "Axis"=w766, "error in"=w773, "VISA in"=w764, "Position (mm or degree)"=w765) -> ("error out"=w772:errorcluster, "VISA out"=w767:refnum<visa-resource-name>)  [unwired: 5 in]
                n576 = call "Motors Move Absolute.vi"("Axis Multiplier"=w754, "Axis"=w768, "error in"=w772, "VISA in"=w767, "Position (mm or degree)"=w769) -> ("error out"=w771:errorcluster, "VISA out"=w770:refnum<visa-resource-name>)  [unwired: 5 in]
              }
            }
            n577 = property on="Need to Update Motor Parameters" class="LVObjRef (strict)"() -> ("Value"=w168:refnum<vi>)  [unwired: 2 in, 2 out]
            n578 = property on="Property Node" class="Bool (strict)"(reference=w168) -> (reference out=w185:refnum<vi>, "Value"=w284:bool)  [unwired: 1 in, 1 out]
            n579 = case shown="True" w284 {
              tunnel: w279 -> [w853 w860]
              tunnel: w278 -> [w852 w861]
              tunnel: [w852 w859] -> w145
              tunnel: [w853 w858] -> w148
              tunnel: w186 -> [_ w857]
              tunnel: w185 -> [_ w856]
              frame False {
              }
              frame True {
                n580 = flat-sequence {
                  tunnel: w857 -> [w864]
                  tunnel: [w863] -> w855
                  tunnel: w861 -> [w899]
                  tunnel: w860 -> [w898]
                  tunnel: [w897] -> w859
                  tunnel: [w896] -> w858
                  tunnel: w855 -> [w890]
                  tunnel: [w890] -> w854
                  tunnel: w854 -> [w945]
                  frame #0 {
                    n581 = call <vilib>:"Set Busy.vi"() -> ()  [unwired: 10 in, 2 out]
                    n582 = property on="Property Node" class="Str"(reference=w864, "Value"="Updating Motor Parameters\nThis Should Take About 5 Seconds" ("Status Theta")) -> (reference out=w863:refnum<vi>)  [unwired: 1 in, 1 out]
                  }
                  frame #1 {
                    n583 = call "Motors Status Verbose.vi"("Axis"=1, "VISA in"=w899, "error in"=w898) -> ("Slew Speed (mm or deg/s)"=w915:dbl, "Jogger Normal Speed (mm or deg/s)"=w916:dbl, "Jogger Fast Speed (mm or deg/s)"=w917:dbl, "Actual Position (mm or deg)"=w932:dbl, "OS"=w906:i32, "Mode"=→"X Action":string, "VISA out"=w921:refnum<visa-resource-name>, "Creep Speed (mm or deg/s)"=w894:dbl, "error out"=w903:errorcluster)  [unwired: 4 in]
                    n584 = property on="X Slew Speed (mm or degree/s)" class="LVObjRef (strict)"() -> ("Value"=w877:refnum<vi>)  [unwired: 2 in, 2 out]
                    n585 = property on="Property Node" class="DigNum (strict)"(reference=w877, "Value"=w915) -> ()  [unwired: 1 in, 2 out]
                    n586 = property on="Property Node" class="DigNum (strict)"(reference=w877, "Minimum"=w894) -> ()  [unwired: 1 in, 2 out]
                    n587 = property on="X Jogger Fast Speed" class="LVObjRef (strict)"() -> ("Value"=w878:refnum<vi>)  [unwired: 2 in, 2 out]
                    n588 = property on="X-Axis (mm)" class="LVObjRef (strict)"() -> ("Value"=w873:refnum<vi>)  [unwired: 2 in, 2 out]
                    n589 = property on="X Jogger Normal Speed" class="LVObjRef (strict)"() -> ("Value"=w879:refnum<vi>)  [unwired: 2 in, 2 out]
                    n590 = property on="Property Node" class="DigNum (strict)"(reference=w879, "Value"=w916) -> ()  [unwired: 1 in, 2 out]
                    n591 = property on="Property Node" class="DigNum (strict)"(reference=w878, "Value"=w917) -> ()  [unwired: 1 in, 2 out]
                    n592 = property on="Property Node" class="DigNum (strict)"(reference=w873, "Value"=w932) -> ()  [unwired: 1 in, 2 out]
                    n593 = call "Motors Status Verbose.vi"("Axis"=2, "VISA in"=w921, "error in"=w903) -> ("Slew Speed (mm or deg/s)"=w918:dbl, "Jogger Normal Speed (mm or deg/s)"=w919:dbl, "Jogger Fast Speed (mm or deg/s)"=w920:dbl, "Actual Position (mm or deg)"=w933:dbl, "OS"=w907:i32, "Mode"=→"Y Action":string, "VISA out"=w922:refnum<visa-resource-name>, "Creep Speed (mm or deg/s)"=w893:dbl, "error out"=w904:errorcluster)  [unwired: 4 in]
                    n594 = call "Motors Decipher Status.vi"("OS"=w906) -> ("Status"=w942:string)
                    n595 = property on="Y Slew Speed (mm or degree/s)" class="LVObjRef (strict)"() -> ("Value"=w874:refnum<vi>)  [unwired: 2 in, 2 out]
                    n596 = property on="Property Node" class="DigNum (strict)"(reference=w874, "Value"=w918) -> ()  [unwired: 1 in, 2 out]
                    n597 = property on="Property Node" class="DigNum (strict)"(reference=w874, "Minimum"=w893) -> ()  [unwired: 1 in, 2 out]
                    n598 = Not Equal?(x=w942, y="Idle") -> (x != y?=w924:bool)
                    n599 = property on="Status X" class="LVObjRef (strict)"() -> ("Value"=w881:refnum<vi>)  [unwired: 2 in, 2 out]
                    n600 = property on="Y Jogger Fast Speed" class="LVObjRef (strict)"() -> ("Value"=w887:refnum<vi>)  [unwired: 2 in, 2 out]
                    n601 = property on="Y-Axis (mm)" class="LVObjRef (strict)"() -> ("Value"=w875:refnum<vi>)  [unwired: 2 in, 2 out]
                    n602 = property on="Y Jogger Normal Speed" class="LVObjRef (strict)"() -> ("Value"=w883:refnum<vi>)  [unwired: 2 in, 2 out]
                    n603 = property on="Property Node" class="Str"(reference=w881, "Value"=w942) -> ()  [unwired: 1 in, 2 out]
                    n604 = property on="Property Node" class="DigNum (strict)"(reference=w883, "Value"=w919) -> ()  [unwired: 1 in, 2 out]
                    n605 = property on="Property Node" class="DigNum (strict)"(reference=w887, "Value"=w920) -> ()  [unwired: 1 in, 2 out]
                    n606 = property on="Property Node" class="DigNum (strict)"(reference=w875, "Value"=w933) -> ()  [unwired: 1 in, 2 out]
                    n607 = call "Motors Status Verbose.vi"("Axis"=3, "VISA in"=w922, "error in"=w904) -> ("Slew Speed (mm or deg/s)"=w931:dbl, "Jogger Normal Speed (mm or deg/s)"=w930:dbl, "Jogger Fast Speed (mm or deg/s)"=w929:dbl, "Actual Position (mm or deg)"=w928:dbl, "OS"=w908:i32, "Mode"=→"Z Action":string, "VISA out"=w923:refnum<visa-resource-name>, "Creep Speed (mm or deg/s)"=w892:dbl, "error out"=w905:errorcluster)  [unwired: 4 in]
                    n608 = call "Motors Decipher Status.vi"("OS"=w907) -> ("Status"=w934:string)
                    n609 = property on="X Moving" class="LVObjRef (strict)"() -> ("Value"=w880:refnum<vi>)  [unwired: 2 in, 2 out]
                    n610 = property on="Z Slew Speed (mm or degree/s)" class="LVObjRef (strict)"() -> ("Value"=w876:refnum<vi>)  [unwired: 2 in, 2 out]
                    n611 = property on="Property Node" class="Bool (strict)"(reference=w880, "Value"=w924) -> ()  [unwired: 1 in, 2 out]
                    n612 = property on="Property Node" class="DigNum (strict)"(reference=w876, "Value"=w931) -> ()  [unwired: 1 in, 2 out]
                    n613 = property on="Property Node" class="DigNum (strict)"(reference=w876, "Minimum"=w892) -> ()  [unwired: 1 in, 2 out]
                    n614 = Not Equal?(x=w934, y="Idle") -> (x != y?=w925:bool)
                    n615 = property on="Status Y" class="LVObjRef (strict)"() -> ("Value"=w870:refnum<vi>)  [unwired: 2 in, 2 out]
                    n616 = property on="Z Jogger Fast Speed" class="LVObjRef (strict)"() -> ("Value"=w885:refnum<vi>)  [unwired: 2 in, 2 out]
                    n617 = property on="Z-Axis (mm)" class="LVObjRef (strict)"() -> ("Value"=w889:refnum<vi>)  [unwired: 2 in, 2 out]
                    n618 = property on="Z Jogger Normal Speed" class="LVObjRef (strict)"() -> ("Value"=w886:refnum<vi>)  [unwired: 2 in, 2 out]
                    n619 = property on="Property Node" class="Str"(reference=w870, "Value"=w934) -> ()  [unwired: 1 in, 2 out]
                    n620 = property on="Property Node" class="DigNum (strict)"(reference=w886, "Value"=w930) -> ()  [unwired: 1 in, 2 out]
                    n621 = property on="Property Node" class="DigNum (strict)"(reference=w885, "Value"=w929) -> ()  [unwired: 1 in, 2 out]
                    n622 = property on="Property Node" class="DigNum (strict)"(reference=w889, "Value"=w928) -> ()  [unwired: 1 in, 2 out]
                    n623 = call "Motors Status Verbose.vi"("Axis"=4, "VISA in"=w923, "error in"=w905) -> ("Slew Speed (mm or deg/s)"=w937:dbl, "Jogger Normal Speed (mm or deg/s)"=w938:dbl, "Jogger Fast Speed (mm or deg/s)"=w939:dbl, "Actual Position (mm or deg)"=w940:dbl, "OS"=w909:i32, "Mode"=→"Theta Action":string, "VISA out"=w897:refnum<visa-resource-name>, "Creep Speed (mm or deg/s)"=w891:dbl, "error out"=w896:errorcluster)  [unwired: 4 in]
                    n624 = call "Motors Decipher Status.vi"("OS"=w908) -> ("Status"=w936:string)
                    n625 = property on="Y Moving" class="LVObjRef (strict)"() -> ("Value"=w888:refnum<vi>)  [unwired: 2 in, 2 out]
                    n626 = property on="Theta Slew Speed (mm or degree/s)" class="LVObjRef (strict)"() -> ("Value"=w867:refnum<vi>)  [unwired: 2 in, 2 out]
                    n627 = property on="Property Node" class="Bool (strict)"(reference=w888, "Value"=w925) -> ()  [unwired: 1 in, 2 out]
                    n628 = property on="Property Node" class="DigNum (strict)"(reference=w867, "Value"=w937) -> ()  [unwired: 1 in, 2 out]
                    n629 = property on="Property Node" class="DigNum (strict)"(reference=w867, "Minimum"=w891) -> ()  [unwired: 1 in, 2 out]
                    n630 = Not Equal?(x=w936, y="Idle") -> (x != y?=w926:bool)
                    n631 = property on="Theta Jogger Fast Speed" class="LVObjRef (strict)"() -> ("Value"=w869:refnum<vi>)  [unwired: 2 in, 2 out]
                    n632 = property on="Theta (deg)" class="LVObjRef (strict)"() -> ("Value"=w872:refnum<vi>)  [unwired: 2 in, 2 out]
                    n633 = property on="Status Z" class="LVObjRef (strict)"() -> ("Value"=w871:refnum<vi>)  [unwired: 2 in, 2 out]
                    n634 = property on="Theta Jogger Normal Speed" class="LVObjRef (strict)"() -> ("Value"=w868:refnum<vi>)  [unwired: 2 in, 2 out]
                    n635 = property on="Property Node" class="Str"(reference=w871, "Value"=w936) -> ()  [unwired: 1 in, 2 out]
                    n636 = property on="Property Node" class="DigNum (strict)"(reference=w868, "Value"=w938) -> ()  [unwired: 1 in, 2 out]
                    n637 = property on="Property Node" class="DigNum (strict)"(reference=w869, "Value"=w939) -> ()  [unwired: 1 in, 2 out]
                    n638 = property on="Property Node" class="DigNum (strict)"(reference=w872, "Value"=w940) -> ()  [unwired: 1 in, 2 out]
                    n639 = call "Motors Decipher Status.vi"("OS"=w909) -> ("Status"=w944:string)
                    n640 = property on="Z Moving" class="LVObjRef (strict)"() -> ("Value"=w882:refnum<vi>)  [unwired: 2 in, 2 out]
                    n641 = property on="Property Node" class="Bool (strict)"(reference=w882, "Value"=w926) -> ()  [unwired: 1 in, 2 out]
                    n642 = Not Equal?(x=w944, y="Idle") -> (x != y?=w927:bool)
                    n643 = property on="Status Theta" class="LVObjRef (strict)"() -> ("Value"=w884:refnum<vi>)  [unwired: 2 in, 2 out]
                    n644 = property on="Property Node" class="Str"(reference=w884, "Value"=w944) -> ()  [unwired: 1 in, 2 out]
                    n645 = property on="Theta Moving" class="LVObjRef (strict)"() -> ("Value"=w866:refnum<vi>)  [unwired: 2 in, 2 out]
                    n646 = property on="Property Node" class="Bool (strict)"(reference=w866, "Value"=w927) -> ()  [unwired: 1 in, 2 out]
                  }
                  frame #2 {
                    n647 = call <vilib>:"Unset Busy.vi"() -> ()  [unwired: 11 in, 1 out]
                    n648 = property on="Property Node" class="Str"(reference=w945, "Value"="Running" ("Status Theta")) -> ()  [unwired: 1 in, 2 out]
                  }
                }
                n649 = property on="Property Node" class="Bool (strict)"(reference=w856, "Value"=FALSE ("Need to Update Motor Parameters")) -> ()  [unwired: 1 in, 2 out]
              }
            }
            n650 = property on="Property Node" class="Clust (strict)"(reference=w147, "Value"=w148) -> ()  [unwired: 1 in, 2 out]
            "Loop i" <- w263
          }
        }
      }
    }
  }
  n651 = property on="Property Node" class="Clust (strict)"(reference=w1) -> (reference out=w17:refnum<vi>, "Value"=w19:errorcluster)  [unwired: 1 in, 1 out]
  n652 = call "Motors Close.vi"("error in"=w19, "VISA in"=w3) -> ("error out"=w18:errorcluster)  [unwired: 1 in]
  n653 = property on="Property Node" class="Clust (strict)"(reference=w17, "Value"=w18) -> ()  [unwired: 1 in, 2 out]
